vi "Calibration.vi"(7 "Show Front Panel":bool=TRUE, 8 "error in (no error)":errorcluster, 11 "file path (dialog if empty)":path=path "C:/work/Calibration.csv") -> (0 "error out":errorcluster, 3 "OutputData":string[][](array[string]))   [LabVIEW 2014]
uses:
  Type Definitions/HEWH Calibration.ctl
  Type Definitions/HEWH CalibrationTime.ctl
  Type Definitions/HEWH Calibration_SN.ctl
  Support VIs/CALIBRATION Equipment.vi
  <vilib>/Utility/file.llb/Write To Spreadsheet File (string).vi
panel:
  out "concatenated string":string
  out "snta":string[](array[string])
  in  "Tab Control":enum32{"Calibration Dates", "File Location"}(tab)
  in  "Equipment Description":T1
  in  "Manufacturer":T1
  in  "Model Number":T1
  in  "Calibration ID":T1
  in  "Complete":bool
  in  "Serial Number":T2
  in  "Last Calibrated":T3 {"Eq20" format="%<%x>T"; "Eq19" format="%<%x>T"; "Eq18" format="%<%x>T"; "Eq17" format="%<%x>T"; "Eq16" format="%<%x>T"; "Eq15" format="%<%x>T"; "Eq14" format="%<%x>T"; "Eq13" format="%<%x>T"; "Eq12" format="%<%x>T"; "Eq11" format="%<%x>T"; "Eq10" format="%<%x>T"; "Eq9" format="%<%x>T"; "Eq8" format="%<%x>T"; "Eq7" format="%<%x>T"; "Eq6" format="%<%x>T"; "Eq5" format="%<%x>T"; "Eq4" format="%<%x>T"; "Eq3" format="%<%x>T"; "Eq2" format="%<%x>T"; "Eq1" format="%<%x>T"}
  in  "Calibration Due":T3 {"Eq20" format="%<%x>T"; "Eq19" format="%<%x>T"; "Eq18" format="%<%x>T"; "Eq17" format="%<%x>T"; "Eq16" format="%<%x>T"; "Eq15" format="%<%x>T"; "Eq14" format="%<%x>T"; "Eq13" format="%<%x>T"; "Eq12" format="%<%x>T"; "Eq11" format="%<%x>T"; "Eq10" format="%<%x>T"; "Eq9" format="%<%x>T"; "Eq8" format="%<%x>T"; "Eq7" format="%<%x>T"; "Eq6" format="%<%x>T"; "Eq5" format="%<%x>T"; "Eq4" format="%<%x>T"; "Eq3" format="%<%x>T"; "Eq2" format="%<%x>T"; "Eq1" format="%<%x>T"}
  in  "Size":i32=20
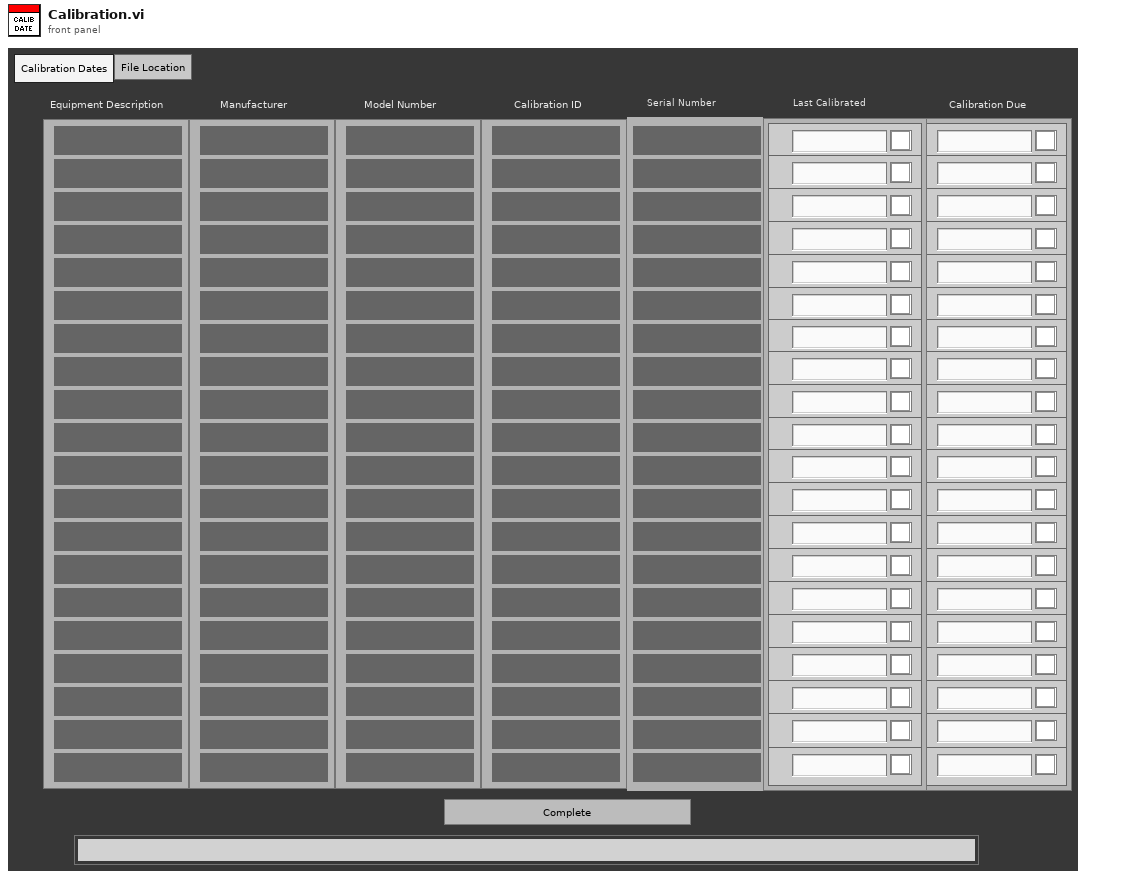
[diagram p1: front panel]
types:
  T1 = typedef "HEWH Calibration.ctl" = cluster{"Eq 1":string, "Eq 2":string, "Eq 3":string, "Eq 4":string, "Eq 5":string, "Eq 6":string, "Eq 7":string, "Eq 8":string, "Eq 9":string, "Eq 10":string, "Eq 11":string, "Eq 12":string, "Eq 13":string, "Eq 14":string, "Eq 15":string, "Eq 16":string, "Eq 17":string, "Eq 18":string, "Eq 19":string, "Eq 20":string}
  T2 = typedef "HEWH Calibration_SN.ctl" = cluster{"Eq 1":string, "Eq 2":string, "Eq 3":string, "Eq 4":string, "Eq 5":string, "Eq 6":string, "Eq 7":string, "Eq 8":string, "Eq 9":string, "Eq 10":string, "Eq 11":string, "Eq 12":string, "Eq 13":string, "Eq 14":string, "Eq 15":string, "Eq 16":string, "Eq 17":string, "Eq 18":string, "Eq 19":string, "Eq 20":string}
  T3 = typedef "HEWH CalibrationTime.ctl" = cluster{"Eq1":timestamp, "Eq2":timestamp, "Eq3":timestamp, "Eq4":timestamp, "Eq5":timestamp, "Eq6":timestamp, "Eq7":timestamp, "Eq8":timestamp, "Eq9":timestamp, "Eq10":timestamp, "Eq11":timestamp, "Eq12":timestamp, "Eq13":timestamp, "Eq14":timestamp, "Eq15":timestamp, "Eq16":timestamp, "Eq17":timestamp, "Eq18":timestamp, "Eq19":timestamp, "Eq20":timestamp}
  T4 = cluster{"Calibration Due":T3, "Last Calibrated":T3, "Serial Number":T2, "Calibration ID":T1, "Model Number":T1, "Manufacturer":T1, "Equipment Description":T1, i32}
  T5 = enum32{"invalid app kind", "Development System", "Run Time System", "Student Edition", "Embedded LabVIEW", "Evaluation", "Custom"}
  T6 = enum32{"Invalid", "Standard", "Closed", "Hidden", "Minimized", "Maximized"}
  T7 = cluster{"Core":cluster{"Current VI Reference":refnum<vi>, "Close Panel on Exit?":bool}, "Calibration Due":T3, "file path (dialog if empty)":path, "Serial Number":T2, "Calibration ID":T1, "Total Array":string[][], "Size":i32, "Last Calibrated":T3, "Model Number":T1, "Manufacturer":T1, "Equipment Description":T1}
  T8 = cluster{"Current VI Reference":refnum<vi>, "Close Panel on Exit?":bool}
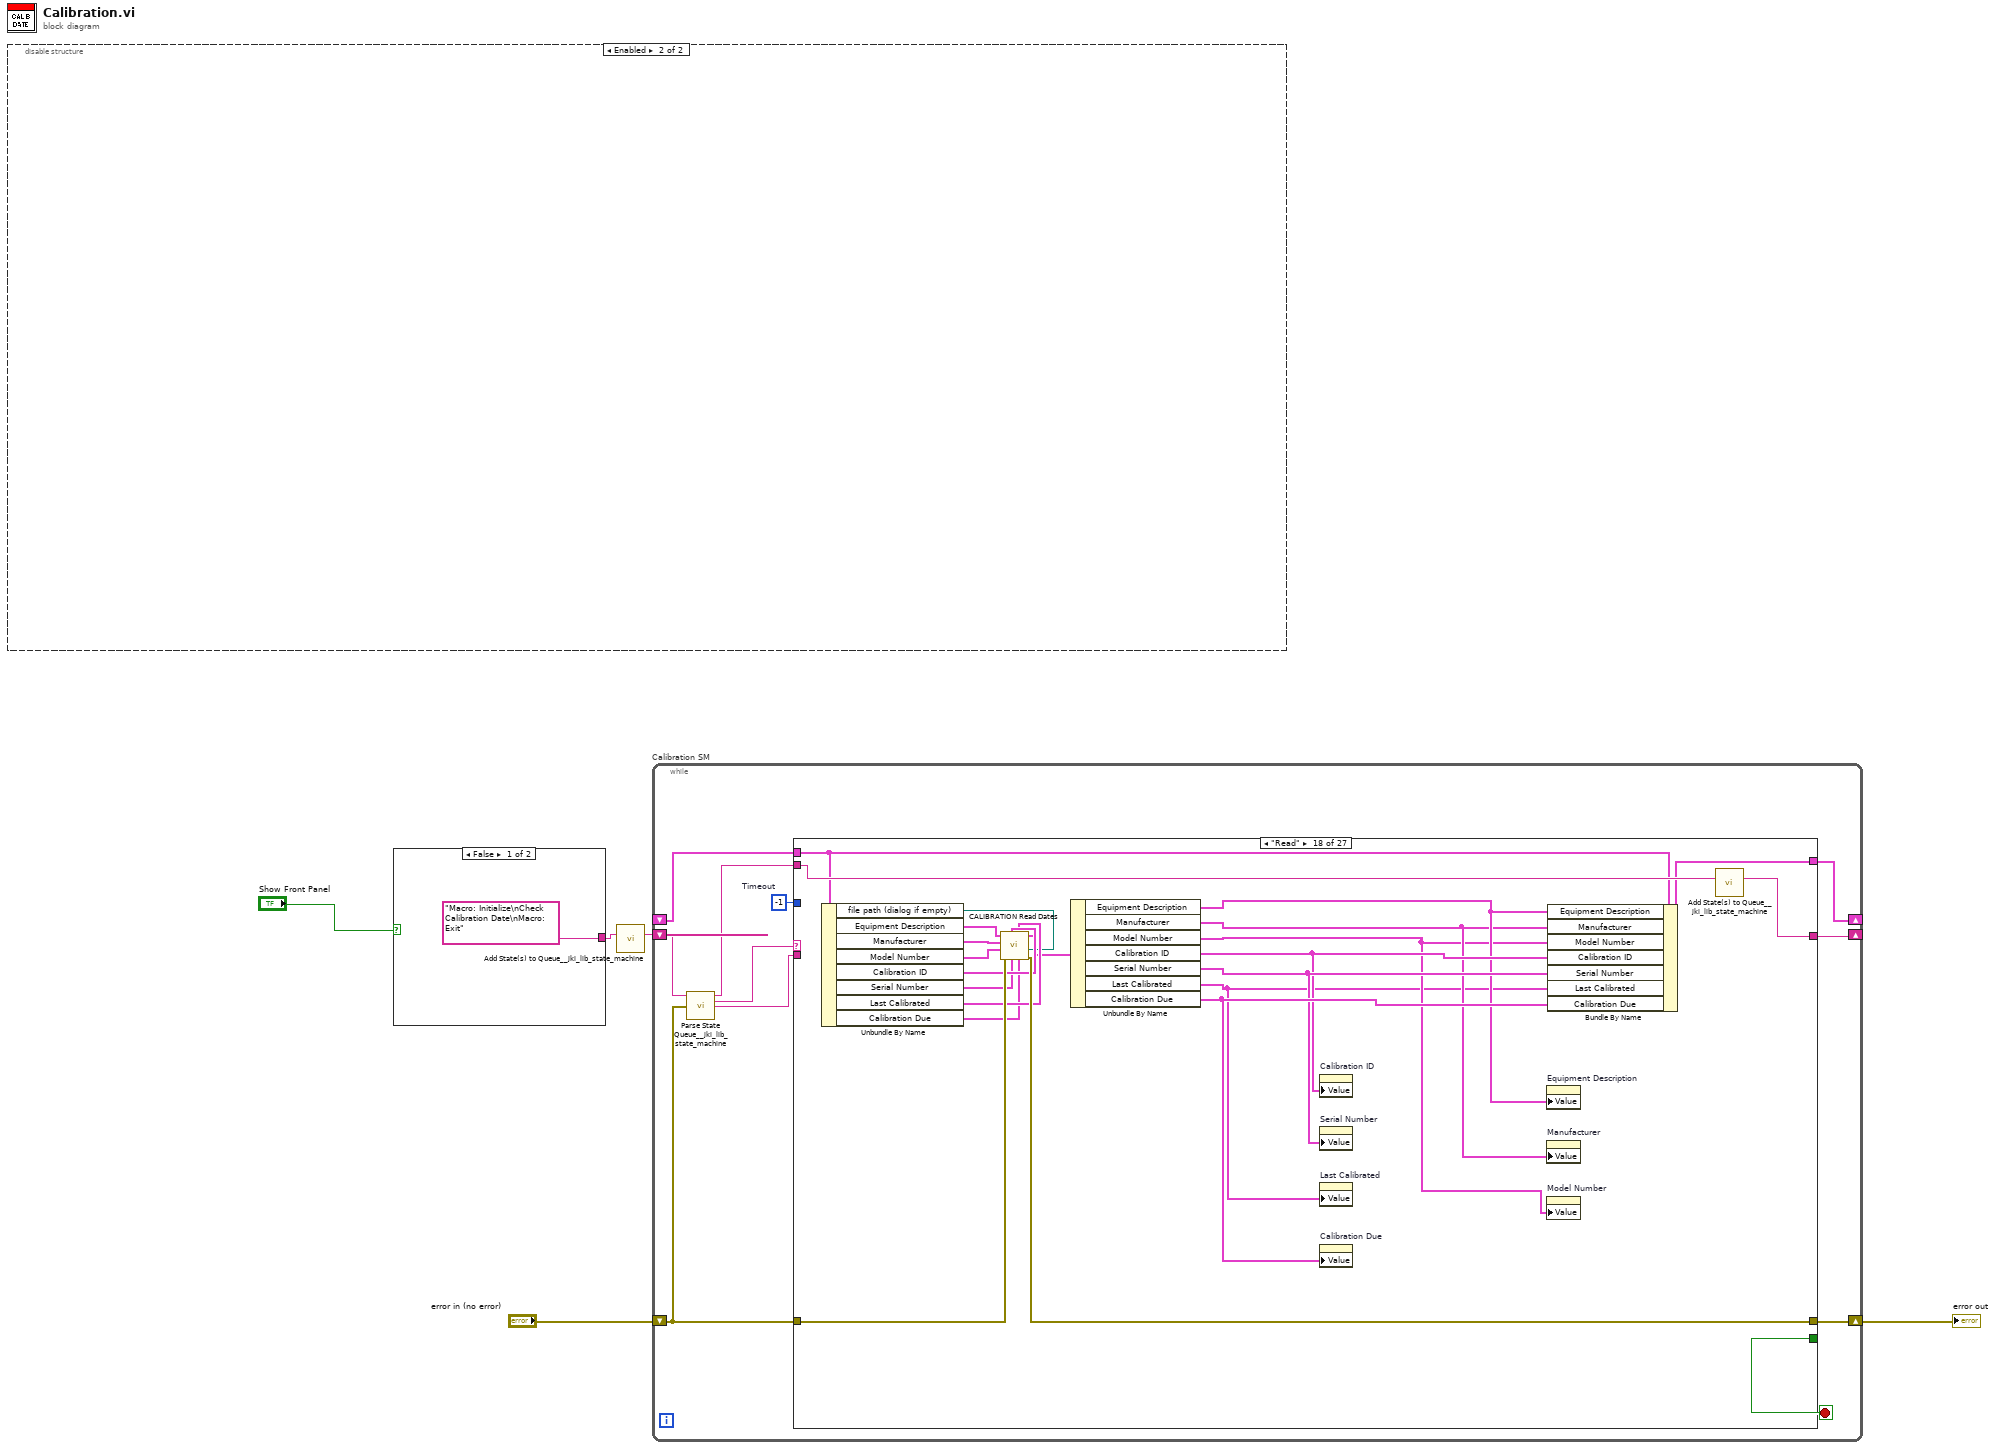
[diagram p0: block diagram]
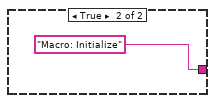
[diagram p2: hidden frame]
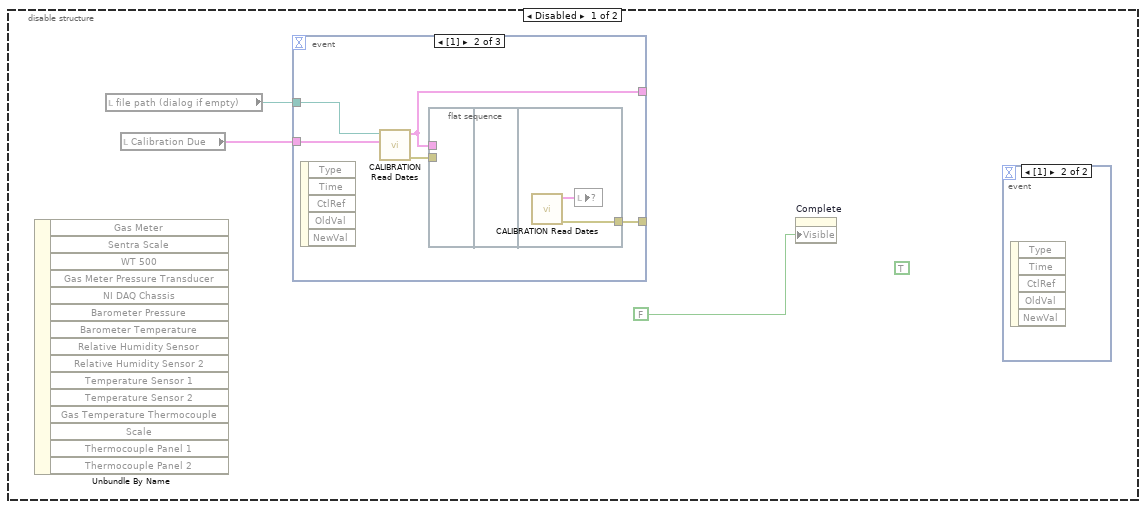
[diagram p3: hidden frame]
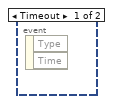
[diagram p4: hidden frame]
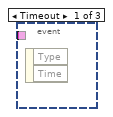
[diagram p5: hidden frame]
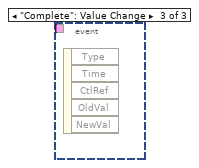
[diagram p6: hidden frame]
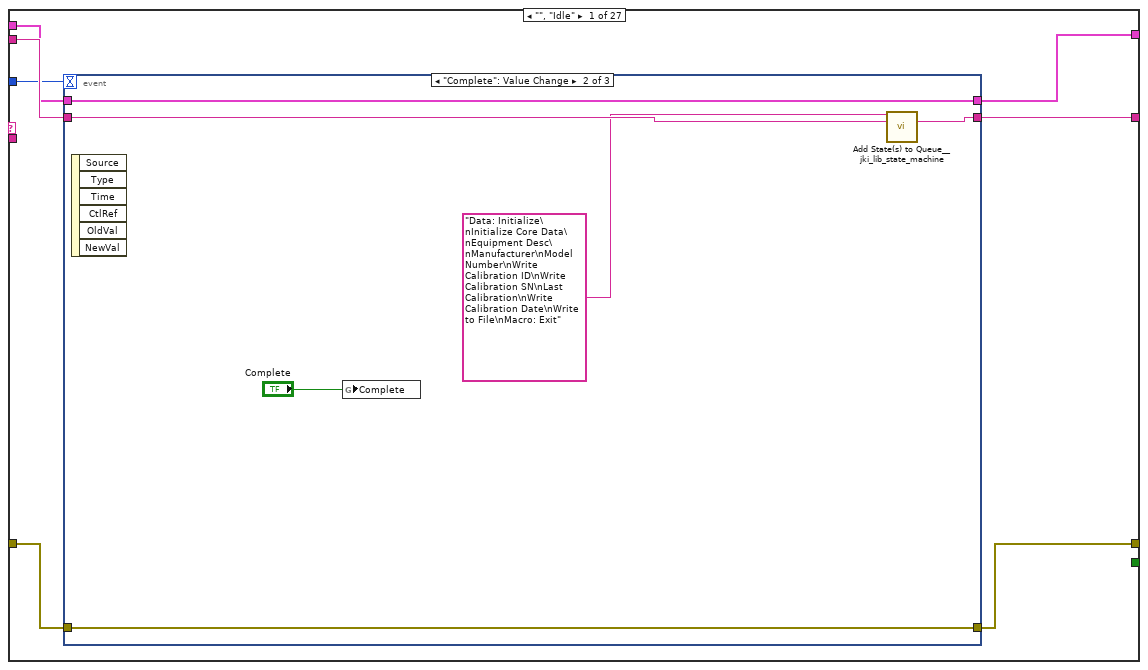
[diagram p7: hidden frame]
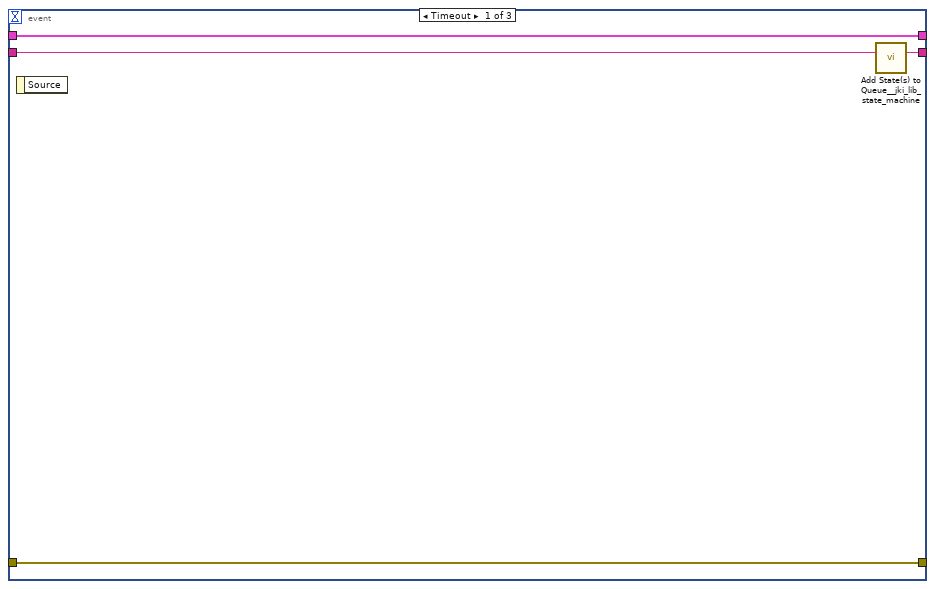
[diagram p8: hidden frame]
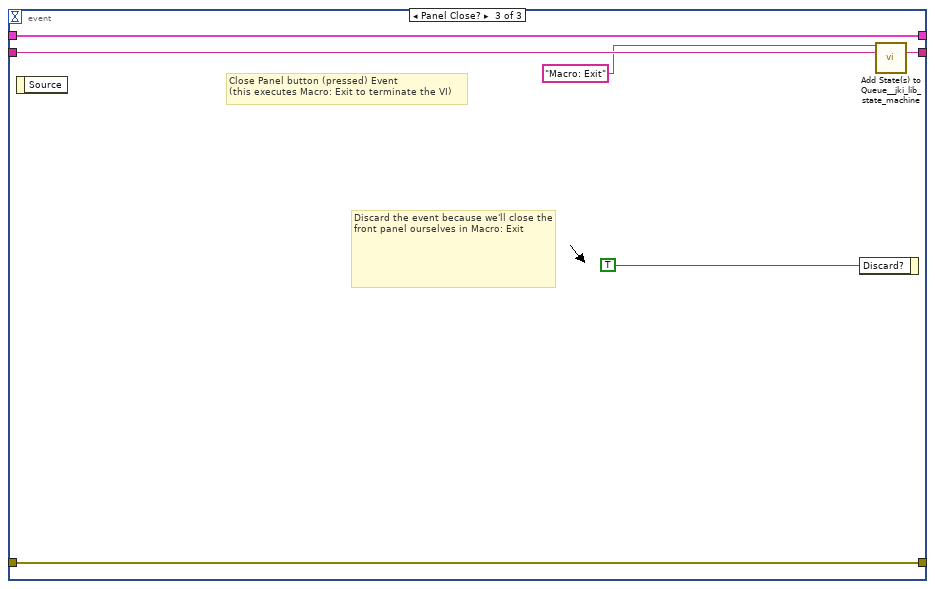
[diagram p9: hidden frame]
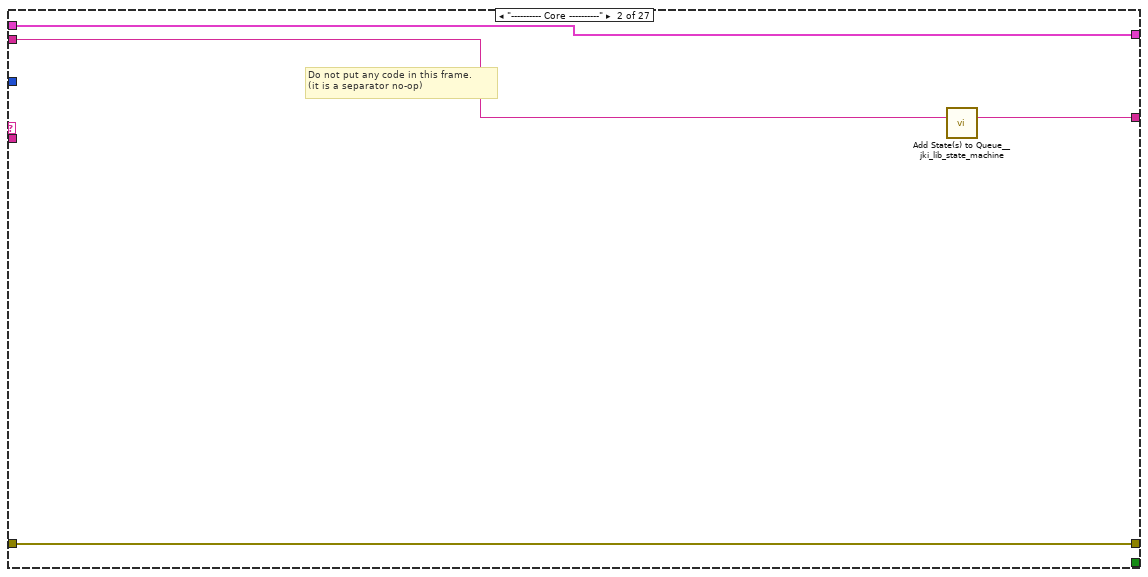
[diagram p10: hidden frame]
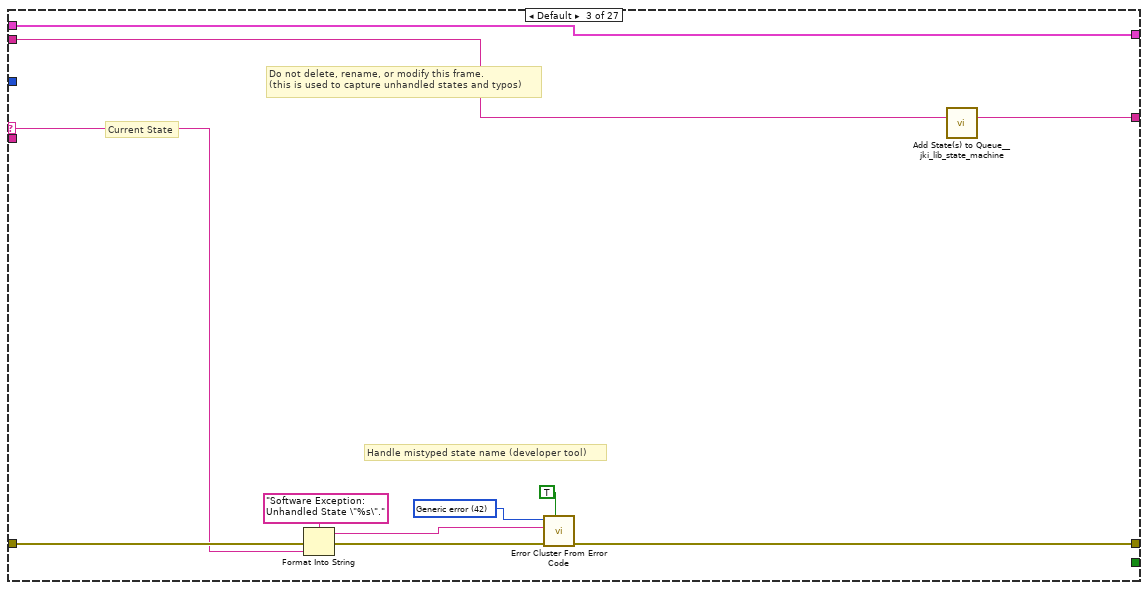
[diagram p11: hidden frame]
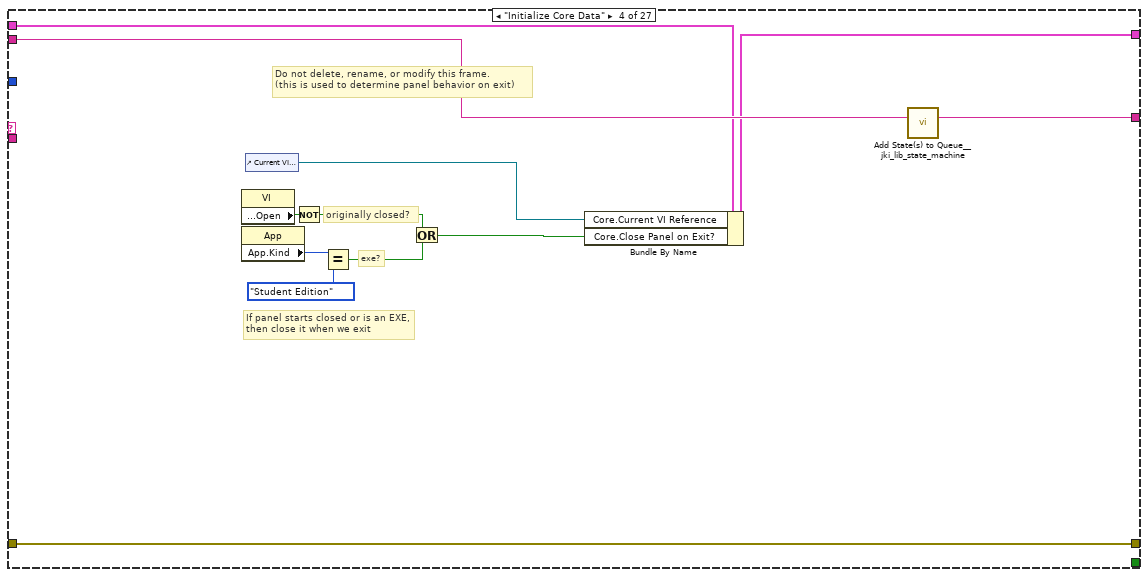
[diagram p12: hidden frame]
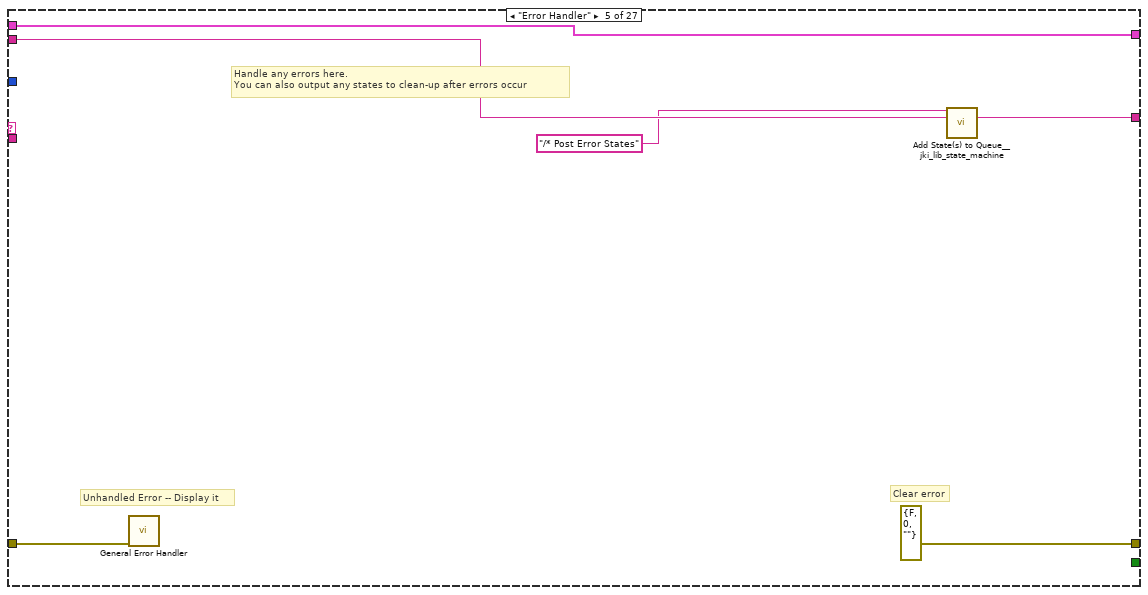
[diagram p13: hidden frame]
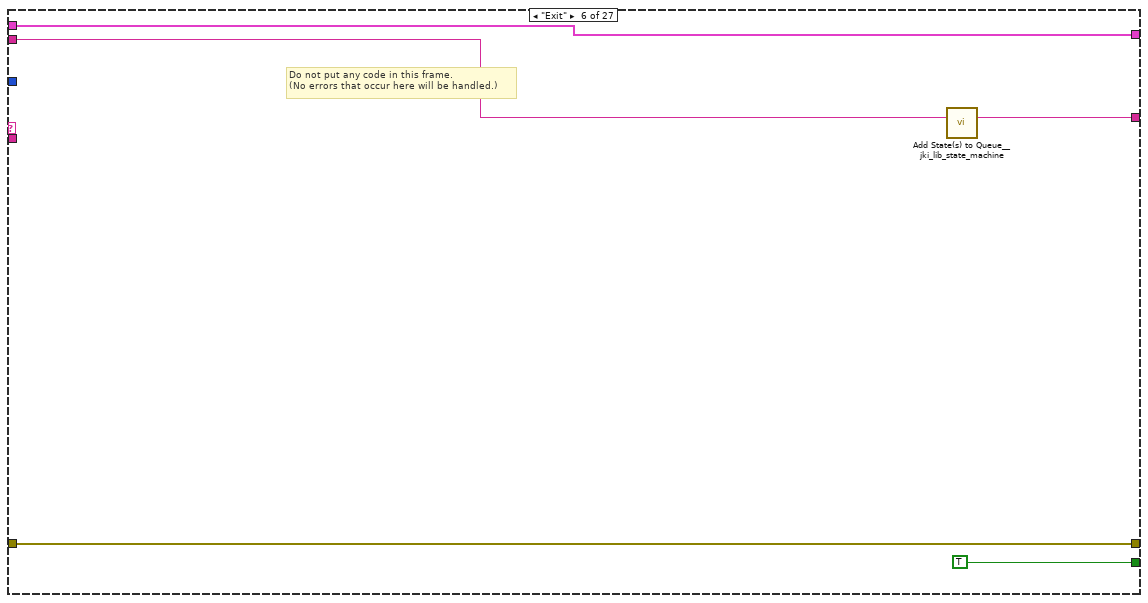
[diagram p14: hidden frame]
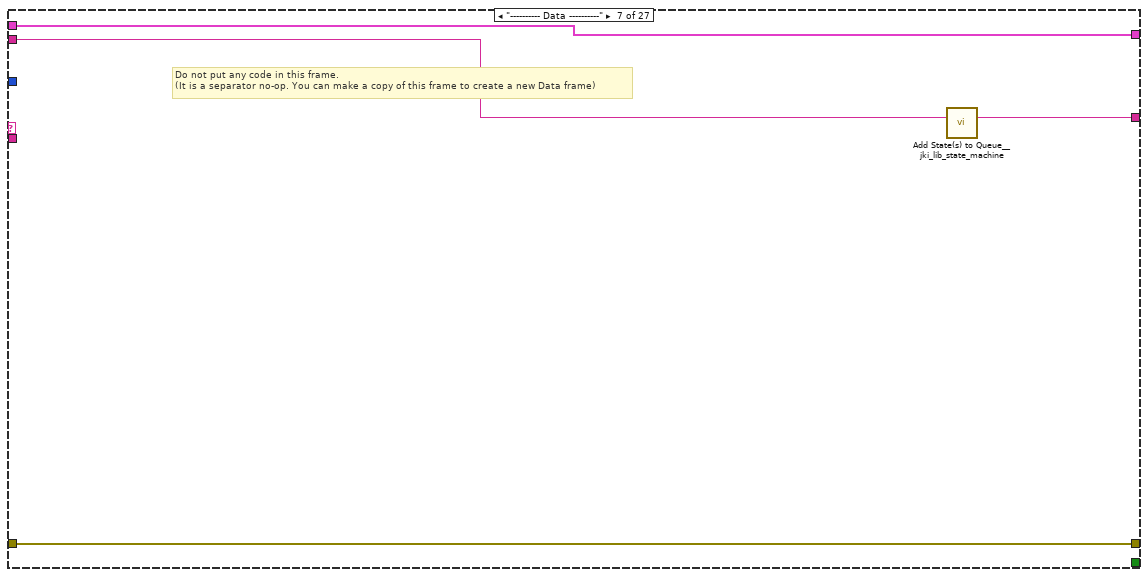
[diagram p15: hidden frame]
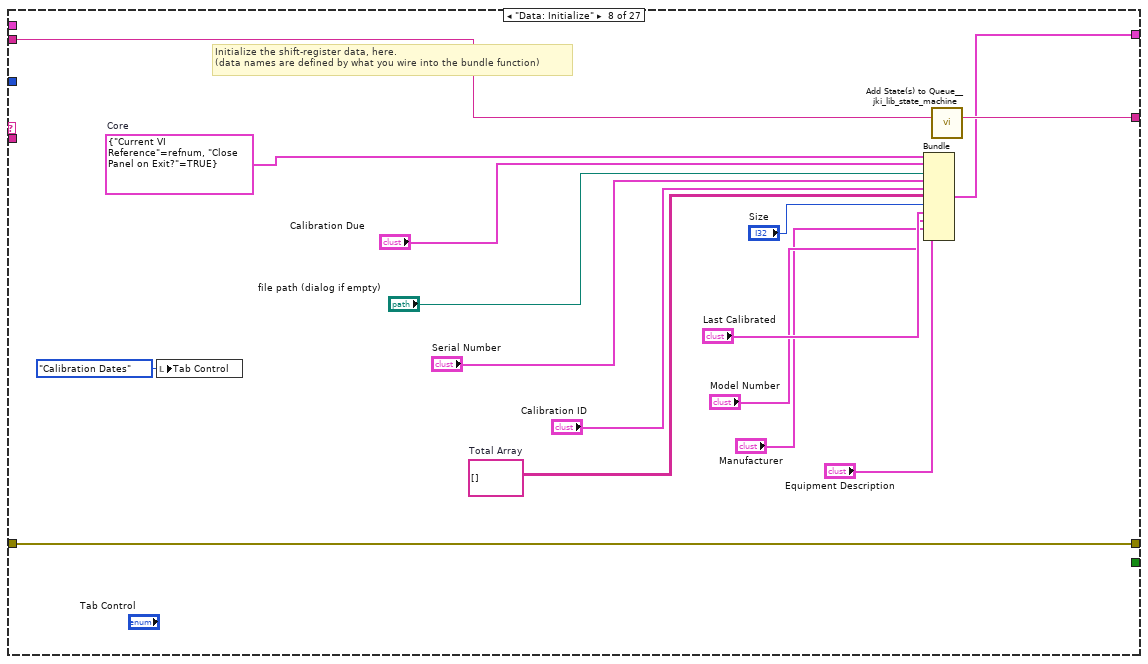
[diagram p16: hidden frame]
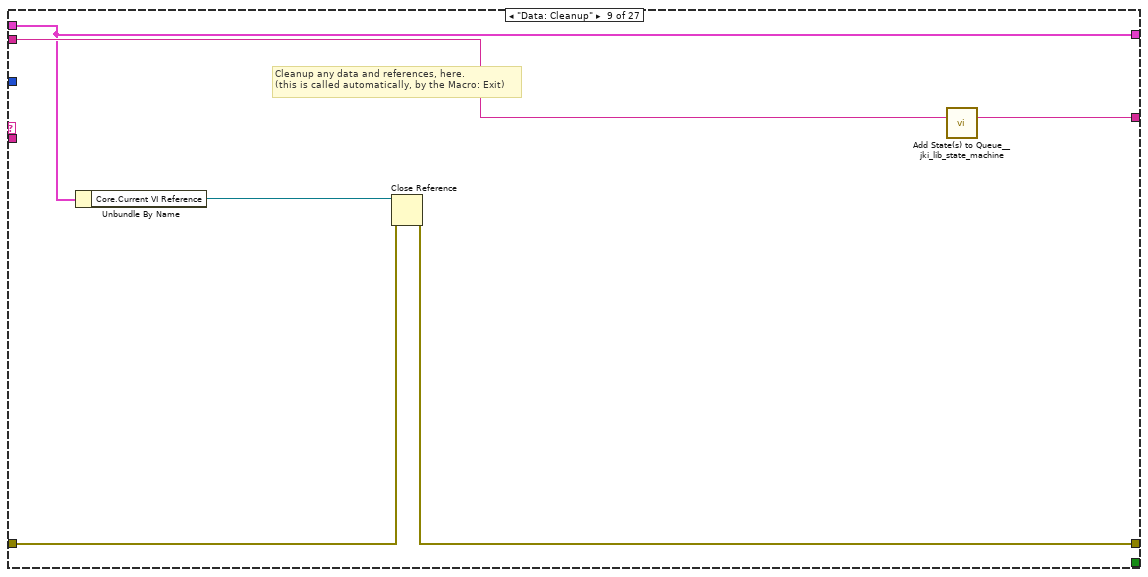
[diagram p17: hidden frame]
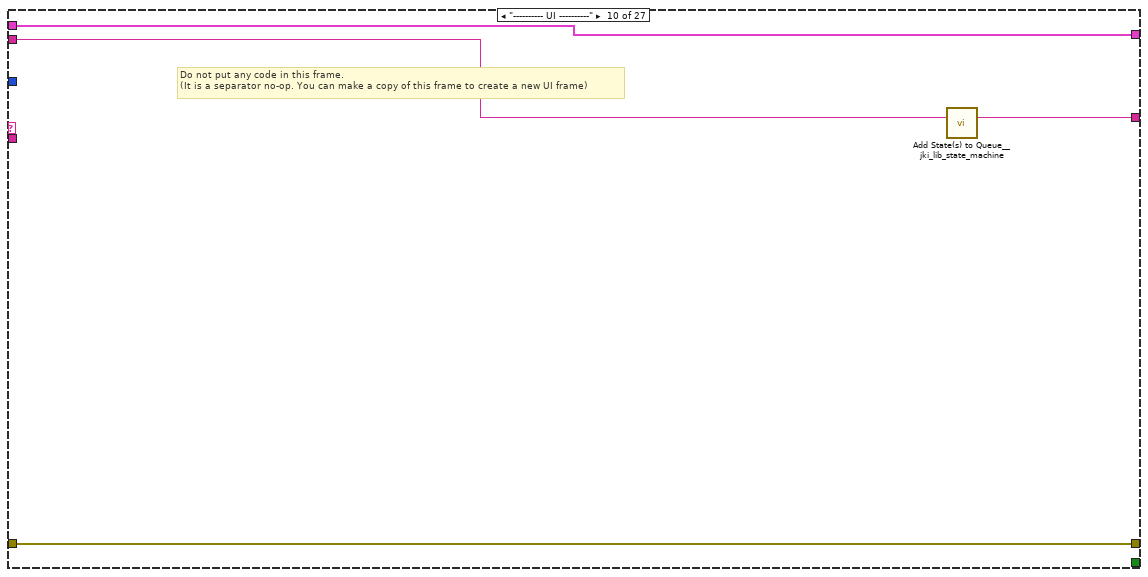
[diagram p18: hidden frame]
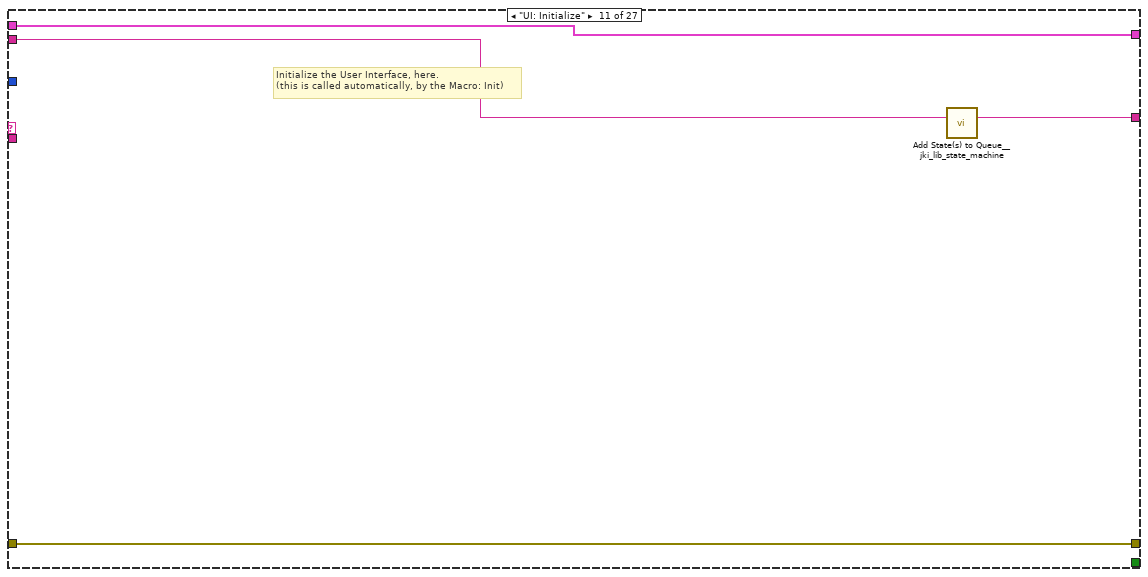
[diagram p19: hidden frame]
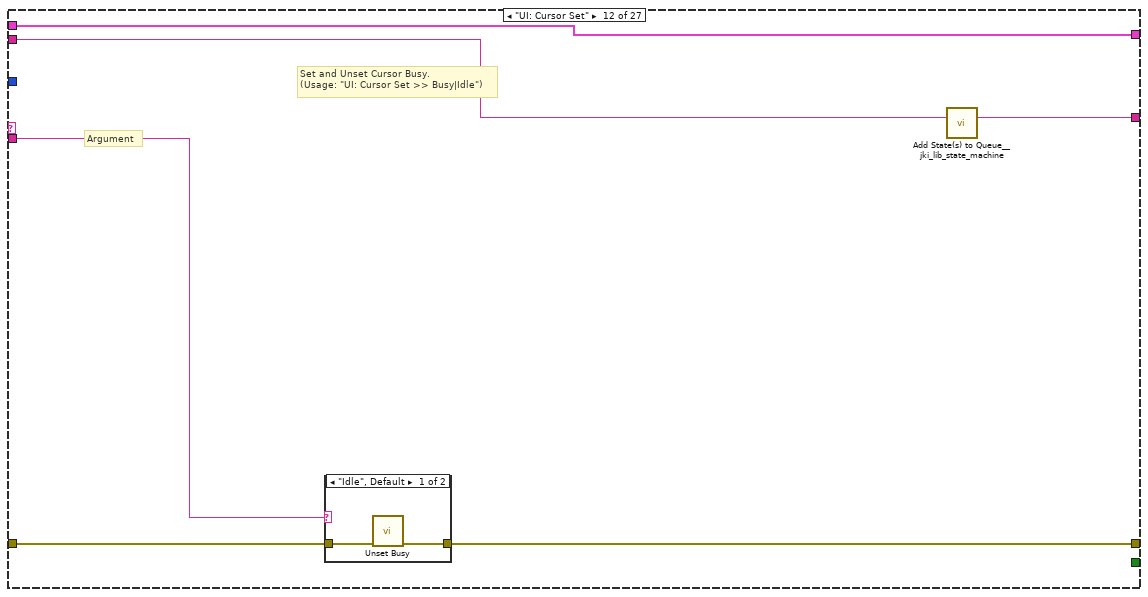
[diagram p20: hidden frame]
diagram:
  n1 = disable-structure shown="Enabled" {
    frame Disabled {
      w8 = TRUE ("Visible")
      n2 = Unbundle By Name() -> ()  [unwired: 1 in, 15 out]
      n3 = local read "file path (dialog if empty)"() -> (w6:path)
      n4 = local read "Calibration Due"() -> (w7:T3)
      n5 = event shown="[1]" {
        selector: _ -> [_ _ _]
        dyn-events: _ -> [_ _ _]
        timeout: _ -> [_ _ _]
        tunnel: [_ w12 _] -> _
        tunnel: [_ w15 _] -> _
        tunnel: w7 -> [_ w14 _]
        tunnel: w6 -> [_ w13 _]
        event Timeout {
          n6 = event-data() -> ()  [unwired: 1 in, 2 out]
        }
        event #1 (no event record) {
          n7 = event-data() -> ()  [unwired: 1 in, 5 out]
          n8 = call "CALIBRATION Read Dates.vi"("Manufacturer"=w14, "Equipment Description"=w13) -> ("error out"=w11:errorcluster, "output cluster"=w12:T4)  [unwired: 8 in]
          n9 = flat-sequence {
            tunnel: w11 -> [_]
            tunnel: w12 -> [_]
            tunnel: [w16] -> w15
            frame #0 {
            }
            frame #1 {
            }
            frame #2 {
              n10 = call "CALIBRATION Read Dates.vi"() -> ("error out"=w16:errorcluster, "output cluster"=w17:T4)  [unwired: 10 in]
              n11 = local write item#-1(w17) -> ()
            }
          }
        }
        event "Complete": Value Change {
          n12 = event-data() -> ()  [unwired: 1 in, 5 out]
        }
      }
      n13 = property on="Complete" class="Bool"("Visible"=FALSE) -> (error out=w9:errorcluster)  [unwired: 2 in, 1 out]
      n14 = event shown="[1]" {
        selector: _ -> [_ _]
        dyn-events: _ -> [_ _]
        timeout: _ -> [_ _]
        event Timeout {
          n15 = event-data() -> ()  [unwired: 1 in, 2 out]
        }
        event #1 (no event record) {
          n16 = event-data() -> ()  [unwired: 1 in, 5 out]
        }
      }
    }
    frame Enabled {
    }
  }
  n17 = case shown="False" "Show Front Panel" {
    tunnel: ["Macro: Initialize\nCheck Calibration Date\nMacro: Exit" "Macro: Initialize"] -> w4
    frame False {
    }
    frame True {
    }
  }
  n18 = call <vilib>:"Add State(s) to Queue__jki_lib_state_machine.vi"("State(s) in (\"\")"=w4) -> ("States Out"=w5:string)  [unwired: 14 in]
  n19 = while "Calibration SM" {
    shift-right: [w23] -> _
    shift-left: _ -> [w22]
    shift-right: [w26] -> w2
    shift-left: "error in (no error)" -> [w20]
    shift-right: [w25] -> _
    shift-left: w5 -> [w27]
    stop <- w24 stop-if-true
    w21 = -1  # Timeout
    n20 = call <vilib>:"Parse State Queue__jki_lib_state_machine.vi"("State Queue"=w27, "Error In (no error)"=w20) -> ("Remaining States"=w29:string, "Current State"=w30:string, "Arguments"=w28:string)  [unwired: 11 in]
    n21 = case shown="\"Read\"" w30 {
      selector: w30 -> [_ _ w58 _ _ _ _ _ _ _ _ _ _ _ _ _ _ _ _ _ _ _ _ _ _ _ _]
      tunnel: w29 -> [w37 w57 w62 w80 w86 w91 w95 w111 w117 w121 w125 w131 w142 w168 w173 w183 w187 w209 w220 w381 w441 w501 w561 w621 w681 w763 w841]
      tunnel: w28 -> [_ _ _ _ _ _ _ _ _ _ _ w126 w136 _ _ _ _ _ _ _ _ _ _ _ _ _ _]
      tunnel: w22 -> [w35 w54 w60 w71 w83 w89 w92 _ w112 w118 w123 w129 w138 w165 w170 w180 w184 w207 w218 w375 w435 w495 w555 w615 w674 w756 w839]
      tunnel: [w34 w55 w64 w77 errorcluster {"status"=FALSE, "code"=0, "source"=""} ("error out") w88 w93 w108 w113 w119 w122 w127 w139 w166 w171 w181 w185 w204 w217 w376 w436 w496 w556 w616 w676 w758 w836] -> w26
      tunnel: w20 -> [w33 w55 w63 w77 w82 w88 w93 w108 w114 w119 w122 w128 w140 w166 w171 w181 w185 w205 w217 w377 w437 w497 w557 w617 w677 w759 w836]
      tunnel: [w36 w56 w61 w79 w85 w90 w94 w110 w116 w120 w124 w130 w141 w167 w172 w182 w186 w208 w219 w380 w440 w500 w560 w620 w680 w762 w840] -> w25
      tunnel: [_ _ _ _ _ TRUE _ _ _ _ _ _ _ _ _ _ _ _ _ _ _ _ _ _ _ _ _] -> w24
      tunnel: [w32 w54 w60 w78 w83 w89 w92 w109 w112 w118 w123 w129 w138 w165 w170 w180 w184 w206 w218 w374 w434 w494 w554 w614 w673 w755 w839] -> w23
      tunnel: w21 -> [w31 _ _ _ _ _ _ _ _ _ _ _ _ _ _ _ _ _ _ _ _ _ _ _ _ _ _]
      frame "", "Idle" {
        n22 = event shown="[1] \"Complete\": Value Change" {
          selector: _ -> [_ _ _]
          dyn-events: _ -> [_ _ _]
          timeout: w31 -> [_ _ _]
          tunnel: w37 -> [w41 w46 w53]
          tunnel: [w40 w47 w52] -> w36
          tunnel: w35 -> [w38 w43 w50]
          tunnel: [w39 w45 w51] -> w34
          tunnel: w33 -> [w39 w45 w51]
          tunnel: [w38 w43 w50] -> w32
          event Timeout {
            n23 = event-data() -> ()  [unwired: 1 in, 1 out]
            n24 = call <vilib>:"Add State(s) to Queue__jki_lib_state_machine.vi"("State(s) in (\"\")"=w41) -> ("States Out"=w40:string)  [unwired: 14 in]
          }
          event "Complete": Value Change {
            n25 = event-data() -> ()  [unwired: 1 in, 6 out]
            n26 = global write "CALIBRATION Equipment.vi" "Complete"("Complete") -> ()
            n27 = call <vilib>:"Add State(s) to Queue__jki_lib_state_machine.vi"("State(s) in Front (\"\")"="Data: Initialize\nInitialize Core Data\nEquipment Desc\nManufacturer\nModel Number\nWrite Calibration ID\nWrite Calibration SN\nLast Calibration\nWrite Calibration Date\nWrite to File\nMacro: Exit", "State(s) in (\"\")"=w46) -> ("States Out"=w47:string)  [unwired: 13 in]
          }
          event Panel Close? {
            # "Discard the event because we'll close the front panel ourselves in Macro: Exit"
            # "Close Panel button (pressed) Event\n(this executes Macro: Exit to terminate the VI)"
            n28 = event-data() -> ()  [unwired: 1 in, 1 out]
            n29 = event-data("Discard?"=TRUE) -> ()  [unwired: 1 in, 1 out]
            n30 = call <vilib>:"Add State(s) to Queue__jki_lib_state_machine.vi"("State(s) in Front (\"\")"="Macro: Exit", "State(s) in (\"\")"=w53) -> ("States Out"=w52:string)  [unwired: 13 in]
          }
        }
      }
      frame "---------- Core ----------" {
        # "Do not put any code in this frame.\n(it is a separator no-op)"
        n31 = call <vilib>:"Add State(s) to Queue__jki_lib_state_machine.vi"("State(s) in (\"\")"=w57) -> ("States Out"=w56:string)  [unwired: 14 in]
      }
      frame Default {
        w67 = 42 items=["No error", "Argument error", "Memory is full", "Out of zone", "End of file", "File already open", "Generic file I/O error", "File not found", "File permission error", "Disk is full", "Duplicate path", "Too many files open", "System feature not enabled", "Resource file not found", "Cannot add resource", "Resource not found", "Image not found", "Image memory error", "Pen does not exist", "Config type invalid", "Config token not found", "Config parse error", "Config memory error", "Bad external code format", "Bad external code offset", "External code not present", "Null window", "Destroy window error", "Null menu", "Print aborted", "Bad print record", "Print driver error", "Windows error during printing", "Memory error during printing", "Print dialog error", "Generic print error", "Invalid device refnum", "Device not found", "Device parameter error", "Device unit error", "Cannot open device", "Device call aborted", "Generic error", "Cancelled by user", "Object ID too low", "Object ID too high", "Object not in heap", "Unknown heap", "Unknown object (invalid DefProc)", "Unknown object (DefProc not in table)", "Message out of range", "Invalid (null) method", "Unknown message", "Manager call not supported", "Bad address", "Network operation in progress", "Network operation timed out", "Connection is busy", "Network attribute not supported", "Network error", "Address in use", "System out of memory", "Connection aborted", "Connection refused", "Not connected", "Already connected", "Connection closed", "Initialization error (interapplication manager)", "Bad occurrence", "Wait on unbound occurrence handler", "Occurrence queue overflow", "Datalog type conflict", "Unused", "Unrecognized type (interapplication manager)", "Memory corrupt", "Failed to make temporary DLL", "Old CIN version", "Drag socket not found", "Failed to load drop-object", "Failed to register OLE object", "Failed to release OLE object", "Format specifier type mismatch", "Unknown format specifier", "Too few format specifiers", "Too many format specifiers", "Scan failed", "Newer CIN version", "Error converting to variant", "Runtime menu error", "Password tampered", "Variant attribute not found", "Incompatible variant data type", "Event data is not available", "Event Store is not present", "Occurrence is not found", "Event Queue is not created", "Event info is not available", "Refnum passed is NULL", "Error retrieving Class GUID", "Error retrieving CoClass GUID", "Error retrieving TypeLib GUID.", "Bad built application magic bytes.", "Specific driver is different from the specific driver associated with the Logical Name.", "There is no session opened to the class driver.", "Max Error", "MAX - Error with config objects", "MAX - Error loading configuration", "MAX - Group not supported"]
        # "Current State"
        # "Do not delete, rename, or modify this frame.\n(this is used to capture unhandled states and typos)"
        # "Handle mistyped state name (developer tool)"
        n32 = Format Into String(format string="Software Exception: Unhandled State \"%s\"." ("message"), error in=w63, w58) -> (resulting string=w66:string, error out=w65:errorcluster)  [unwired: 1 in]
        n33 = call <vilib>:"Error Cluster From Error Code.vi"("show call chain? (False)"=TRUE, "error in (no error)"=w65, "error message (\"\")"=w66, "error code (0)"=w67) -> ("error out"=w64:errorcluster)  [unwired: 5 in]
        n34 = call <vilib>:"Add State(s) to Queue__jki_lib_state_machine.vi"("State(s) in (\"\")"=w62) -> ("States Out"=w61:string)  [unwired: 14 in]
      }
      frame "Initialize Core Data" {
        # "Do not delete, rename, or modify this frame.\n(this is used to determine panel behavior on exit)"
        # "originally closed?"
        # "exe?"
        # "If panel starts closed or is an EXE, then close it when we exit"
        n35 = property class="VI"() -> ("Front Panel.Open"=w76:bool)  [unwired: 2 in, 2 out]
        n36 = property class="App"() -> ("App.Kind"=w75:T5)  [unwired: 2 in, 2 out]
        n37 = control-ref of="Current VI Reference"() -> (w69:refnum<vi>)
        n38 = Not(x=w76) -> (.not. x?=w73:bool)
        n39 = Equal?(x=w75, y=T5."Student Edition" ("Application:Kind")) -> (x = y?=w72:bool)
        n40 = Or(x=w73, y=w72) -> (x .or. y?=w70:bool)
        n41 = Bundle By Name(cluster=w71, "Core.Current VI Reference"=w69, "Core.Close Panel on Exit?"=w70) -> (w78:T7)
        n42 = call <vilib>:"Add State(s) to Queue__jki_lib_state_machine.vi"("State(s) in (\"\")"=w80) -> ("States Out"=w79:string)  [unwired: 14 in]
      }
      frame "Error Handler" {
        # "Unhandled Error -- Display it"
        # "Handle any errors here.\nYou can also output any states to clean-up after errors occur"
        # "Clear error"
        n43 = call <vilib>:"General Error Handler.vi"("error in (no error)"=w82) -> ()  [unwired: 10 in, 5 out]
        n44 = call <vilib>:"Add State(s) to Queue__jki_lib_state_machine.vi"("State(s) in Front (\"\")"="/* Post Error States", "State(s) in (\"\")"=w86) -> ("States Out"=w85:string)  [unwired: 13 in]
      }
      frame "Exit" {
        # "Do not put any code in this frame.\n(No errors that occur here will be handled.)"
        n45 = call <vilib>:"Add State(s) to Queue__jki_lib_state_machine.vi"("State(s) in (\"\")"=w91) -> ("States Out"=w90:string)  [unwired: 14 in]
      }
      frame "---------- Data ----------" {
        # "Do not put any code in this frame.\n(It is a separator no-op. You can make a copy of this frame to create a new Data frame)"
        n46 = call <vilib>:"Add State(s) to Queue__jki_lib_state_machine.vi"("State(s) in (\"\")"=w95) -> ("States Out"=w94:string)  [unwired: 14 in]
      }
      frame "Data: Initialize" {
        w105 = string[][] []  # Total Array
        w107 = T8 {"Current VI Reference"=refnum, "Close Panel on Exit?"=TRUE}  # Core
        # "Initialize the shift-register data, here.\n(data names are defined by what you wire into the bundle function)"
        n47 = local write "Tab Control"(enum32{"Calibration Dates", "File Location"}."Calibration Dates" ("Tab Control")) -> ()
        n48 = Bundle("Core"=w107, "Calibration Due"="Calibration Due", "file path (dialog if empty)"="file path (dialog if empty)", "Serial Number"="Serial Number", "Calibration ID"="Calibration ID", "Total Array"=w105, "Size"="Size", "Last Calibrated"="Last Calibrated", "Model Number"="Model Number", "Manufacturer"="Manufacturer", "Equipment Description"="Equipment Description") -> (w109:T7)  [unwired: 1 in]
        n49 = call <vilib>:"Add State(s) to Queue__jki_lib_state_machine.vi"("State(s) in (\"\")"=w111) -> ("States Out"=w110:string)  [unwired: 14 in]
      }
      frame "Data: Cleanup" {
        # "Cleanup any data and references, here.\n(this is called automatically, by the Macro: Exit)"
        n50 = Unbundle By Name(w112) -> ("Core.Current VI Reference"=w115:refnum<vi>)
        n51 = Close Reference(reference=w115, error in (no error)=w114) -> (error out=w113:errorcluster)
        n52 = call <vilib>:"Add State(s) to Queue__jki_lib_state_machine.vi"("State(s) in (\"\")"=w117) -> ("States Out"=w116:string)  [unwired: 14 in]
      }
      frame "---------- UI ----------" {
        # "Do not put any code in this frame.\n(It is a separator no-op. You can make a copy of this frame to create a new UI frame)"
        n53 = call <vilib>:"Add State(s) to Queue__jki_lib_state_machine.vi"("State(s) in (\"\")"=w121) -> ("States Out"=w120:string)  [unwired: 14 in]
      }
      frame "UI: Initialize" {
        # "Initialize the User Interface, here.\n(this is called automatically, by the Macro: Init)"
        n54 = call <vilib>:"Add State(s) to Queue__jki_lib_state_machine.vi"("State(s) in (\"\")"=w125) -> ("States Out"=w124:string)  [unwired: 14 in]
      }
      frame "UI: Cursor Set" {
        # "Argument"
        # "Set and Unset Cursor Busy.\n(Usage: \"UI: Cursor Set >> Busy|Idle\")"
        n55 = case shown="\"Idle\", Default" w126 {
          tunnel: w128 -> [w133 w135]
          tunnel: [w132 w134] -> w127
          frame "Idle", Default {
            n56 = call <vilib>:"Unset Busy.vi"("error in (no error)"=w133) -> ("error out"=w132:errorcluster)  [unwired: 10 in]
          }
          frame "Busy" {
            n57 = call <vilib>:"Set Busy.vi"("error in (no error)"=w135) -> ("error out"=w134:errorcluster)  [unwired: 9 in, 1 out]
          }
        }
        n58 = call <vilib>:"Add State(s) to Queue__jki_lib_state_machine.vi"("State(s) in (\"\")"=w131) -> ("States Out"=w130:string)  [unwired: 14 in]
      }
      frame "UI: Front Panel State" {
        # "Argument"
        # "Set Front Panel Open or Closed\n(Usage: \"UI: Front Panel State >> Open|Close\")"
        n59 = Unbundle By Name(w138) -> ("Core.Current VI Reference"=w137:refnum<vi>)
        n60 = case shown="\"Open\", Default" w136 {
          tunnel: w140 -> [w146 w159]
          tunnel: [w148 w160] -> w139
          tunnel: w137 -> [w147 w157]
          frame "Open", Default {
            n61 = property class="VI"(reference=w147, error in=w146) -> (reference out=w144:refnum<vi>, error out=w145:errorcluster, "Front Panel.Open"=w143:bool)
            n62 = case shown="True" w143 {
              tunnel: [w151 w154] -> w148
              tunnel: w145 -> [w150 w154]
              tunnel: w144 -> [w149 _]
              frame False {
                n63 = invoke class="VI" method="FP.Open"(reference=w149, error in=w150, "Activate"=TRUE, "State"=T6."Standard") -> (error out=w151:errorcluster)  [unwired: 1 in, 4 out]
              }
              frame True {
              }
            }
          }
          frame "Close" {
            n64 = property class="VI"(reference=w157, error in=w159) -> (reference out=w156:refnum<vi>, error out=w158:errorcluster, "Front Panel.Open"=w155:bool)
            n65 = case shown="True" w155 {
              tunnel: [w161 w164] -> w160
              tunnel: w158 -> [w161 w163]
              tunnel: w156 -> [_ w162]
              frame False {
              }
              frame True {
                n66 = invoke class="VI" method="FP.Close"(reference=w162, error in=w163) -> (error out=w164:errorcluster)  [unwired: 1 in, 2 out]
              }
            }
          }
        }
        n67 = call <vilib>:"Add State(s) to Queue__jki_lib_state_machine.vi"("State(s) in (\"\")"=w142) -> ("States Out"=w141:string)  [unwired: 14 in]
      }
      frame "---------- Macro ----------" {
        # "Do not put any code in this frame.\n(It is a separator no-op. You can make a copy of this frame to create a new Macro frame)"
        n68 = call <vilib>:"Add State(s) to Queue__jki_lib_state_machine.vi"("State(s) in (\"\")"=w168) -> ("States Out"=w167:string)  [unwired: 14 in]
      }
      frame "Macro: Initialize" {
        w169 = "Data: Initialize\nInitialize Core Data\nUI: Initialize\nUI: Front Panel State >> Open\nRead\nCheck Calibration Date"  # Data: Initialize Initialize Core Data UI: Initialize UI: Front Panel State >> Open Read Check Calibration Date
        # "Initialization Macro\n(This is called once, when the VI starts)"
        n69 = call <vilib>:"Add State(s) to Queue__jki_lib_state_machine.vi"("State(s) in Front (\"\")"=w169, "State(s) in (\"\")"=w173) -> ("States Out"=w172:string)  [unwired: 13 in]
      }
      frame "Macro: Exit" {
        # "Exit Macro\n(This is called once, when the VI exits)"
        n70 = Unbundle By Name(w180) -> ("Core.Close Panel on Exit?"=w179:bool)
        n71 = Select(t="UI: Front Panel State >> Close", s=w179, f="") -> (s? t:f=w176:string)
        n72 = call <vilib>:"Add State(s) to Queue__jki_lib_state_machine.vi"("State(s) in (\"\")"=w176, "State(s) at Back (\"\")"="Data: Cleanup\nExit") -> ("States Out"=w174:string)  [unwired: 13 in]
        n73 = call <vilib>:"Add State(s) to Queue__jki_lib_state_machine.vi"("State(s) in Front (\"\")"=w174, "State(s) in (\"\")"=w183) -> ("States Out"=w182:string)  [unwired: 13 in]
      }
      frame "---------- New Category ----------" {
        # "Template Separator\n(You can make a copy of, or modify, this frame)"
        n74 = call <vilib>:"Add State(s) to Queue__jki_lib_state_machine.vi"("State(s) in (\"\")"=w187) -> ("States Out"=w186:string)  [unwired: 14 in]
      }
      frame "Read" {
        n75 = Unbundle By Name(w207) -> ("file path (dialog if empty)"=w196:path, "Equipment Description"=w203:T1, "Manufacturer"=w202:T1, "Model Number"=w201:T1, "Calibration ID"=w200:T1, "Serial Number"=w199:T2, "Last Calibrated"=w198:T3, "Calibration Due"=w197:T3)
        n76 = call "CALIBRATION Read Dates.vi"("File Path"=w196, "Calibration Due"=w197, "Last Calibrated"=w198, "Serial Number"=w199, "Calibration ID"=w200, "error in (no error)"=w205, "Model Number"=w201, "Manufacturer"=w202, "Equipment Description"=w203) -> ("error out"=w204:errorcluster, "output cluster"=w195:T4)  [unwired: 1 in]
        n77 = Unbundle By Name(w195) -> ("Equipment Description"=w191:T1, "Manufacturer"=w190:T1, "Model Number"=w189:T1, "Calibration ID"=w192:T1, "Serial Number"=w193:T2, "Last Calibrated"=w188:T3, "Calibration Due"=w194:T3)
        n78 = property on="Calibration ID" class="Clust (strict)"("Value"=w192) -> ()  [unwired: 2 in, 2 out]
        n79 = property on="Serial Number" class="Clust (strict)"("Value"=w193) -> ()  [unwired: 2 in, 2 out]
        n80 = property on="Last Calibrated" class="Clust (strict)"("Value"=w188) -> ()  [unwired: 2 in, 2 out]
        n81 = property on="Calibration Due" class="Clust (strict)"("Value"=w194) -> ()  [unwired: 2 in, 2 out]
        n82 = property on="Equipment Description" class="Clust (strict)"("Value"=w191) -> ()  [unwired: 2 in, 2 out]
        n83 = property on="Manufacturer" class="Clust (strict)"("Value"=w190) -> ()  [unwired: 2 in, 2 out]
        n84 = property on="Model Number" class="Clust (strict)"("Value"=w189) -> ()  [unwired: 2 in, 2 out]
        n85 = Bundle By Name(cluster=w207, "Equipment Description"=w191, "Manufacturer"=w190, "Model Number"=w189, "Calibration ID"=w192, "Serial Number"=w193, "Last Calibrated"=w188, "Calibration Due"=w194) -> (w206:T7)
        n86 = call <vilib>:"Add State(s) to Queue__jki_lib_state_machine.vi"("State(s) in (\"\")"=w209) -> ("States Out"=w208:string)  [unwired: 14 in]
      }
      frame "Check Calibration Date" {
        # "Your code here.\n(You can make a copy of, or modify, this frame)"
        n87 = Unbundle By Name(w218) -> ("Calibration Due"=w210:T3, "Size"=w216:i32)
        n88 = for {
          N: w216 -> [_]
          tunnel: w210 -> [w227]
          tunnel: [w225] -> w215 mode=indexing
          i -> [w226]
          n89 = case shown="3" w226 {
            tunnel: w227 -> [w234 w241 w248 w255 w262 w269 w276 w283 w290 w297 w304 w311 w318 w325 w332 w339 w346 w353 w360 w367]
            tunnel: [w228 w235 w243 w249 w256 w263 w270 w277 w284 w291 w299 w306 w313 w319 w327 w334 w341 w348 w354 w361] -> w225
            frame 0, Default {
              n90 = Get Date/Time In Seconds() -> (seconds since 1Jan1904=w233:timestamp)
              n91 = Unbundle By Name(w234) -> ("Eq1"=w232:timestamp)
              n92 = Get Date/Time String(seconds (now)=w233) -> (date string=w231:string)  [unwired: 2 in, 1 out]
              n93 = Get Date/Time String(seconds (now)=w232) -> (date string=w230:string)  [unwired: 2 in, 1 out]
              n94 = call "UTILITY Date String Days.vi"("First date"=w231, "Second date"=w230) -> ("Elapsed days"=w229:i32)  [unwired: 8 in, 1 out]
              n95 = call "HEWH Check for Uninitialized Dates.vi"("date string"=w230, "Elapsed days in"=w229) -> ("Elapsed days out"=w228:i32)  [unwired: 9 in]
            }
            frame 1 {
              n96 = Unbundle By Name(w241) -> ("Eq2"=w238:timestamp)
              n97 = Get Date/Time In Seconds() -> (seconds since 1Jan1904=w240:timestamp)
              n98 = Get Date/Time String(seconds (now)=w240) -> (date string=w239:string)  [unwired: 2 in, 1 out]
              n99 = Get Date/Time String(seconds (now)=w238) -> (date string=w237:string)  [unwired: 2 in, 1 out]
              n100 = call "UTILITY Date String Days.vi"("First date"=w239, "Second date"=w237) -> ("Elapsed days"=w236:i32)  [unwired: 8 in, 1 out]
              n101 = call "HEWH Check for Uninitialized Dates.vi"("date string"=w237, "Elapsed days in"=w236) -> ("Elapsed days out"=w235:i32)  [unwired: 9 in]
            }
            frame 2 {
              n102 = Get Date/Time In Seconds() -> (seconds since 1Jan1904=w247:timestamp)
              n103 = Unbundle By Name(w248) -> ("Eq3"=w245:timestamp)
              n104 = Get Date/Time String(seconds (now)=w247) -> (date string=w246:string)  [unwired: 2 in, 1 out]
              n105 = Get Date/Time String(seconds (now)=w245) -> (date string=w242:string)  [unwired: 2 in, 1 out]
              n106 = call "UTILITY Date String Days.vi"("First date"=w246, "Second date"=w242) -> ("Elapsed days"=w244:i32)  [unwired: 8 in, 1 out]
              n107 = call "HEWH Check for Uninitialized Dates.vi"("date string"=w242, "Elapsed days in"=w244) -> ("Elapsed days out"=w243:i32)  [unwired: 9 in]
            }
            frame 3 {
              n108 = Get Date/Time In Seconds() -> (seconds since 1Jan1904=w254:timestamp)
              n109 = Unbundle By Name(w255) -> ("Eq4"=w252:timestamp)
              n110 = Get Date/Time String(seconds (now)=w254) -> (date string=w253:string)  [unwired: 2 in, 1 out]
              n111 = Get Date/Time String(seconds (now)=w252) -> (date string=w251:string)  [unwired: 2 in, 1 out]
              n112 = call "UTILITY Date String Days.vi"("First date"=w253, "Second date"=w251) -> ("Elapsed days"=w250:i32)  [unwired: 8 in, 1 out]
              n113 = call "HEWH Check for Uninitialized Dates.vi"("date string"=w251, "Elapsed days in"=w250) -> ("Elapsed days out"=w249:i32)  [unwired: 9 in]
            }
            frame 4 {
              n114 = Get Date/Time In Seconds() -> (seconds since 1Jan1904=w261:timestamp)
              n115 = Unbundle By Name(w262) -> ("Eq5"=w259:timestamp)
              n116 = Get Date/Time String(seconds (now)=w261) -> (date string=w260:string)  [unwired: 2 in, 1 out]
              n117 = Get Date/Time String(seconds (now)=w259) -> (date string=w258:string)  [unwired: 2 in, 1 out]
              n118 = call "UTILITY Date String Days.vi"("First date"=w260, "Second date"=w258) -> ("Elapsed days"=w257:i32)  [unwired: 8 in, 1 out]
              n119 = call "HEWH Check for Uninitialized Dates.vi"("date string"=w258, "Elapsed days in"=w257) -> ("Elapsed days out"=w256:i32)  [unwired: 9 in]
            }
            frame 5 {
              n120 = Get Date/Time In Seconds() -> (seconds since 1Jan1904=w268:timestamp)
              n121 = Unbundle By Name(w269) -> ("Eq6"=w266:timestamp)
              n122 = Get Date/Time String(seconds (now)=w268) -> (date string=w267:string)  [unwired: 2 in, 1 out]
              n123 = Get Date/Time String(seconds (now)=w266) -> (date string=w265:string)  [unwired: 2 in, 1 out]
              n124 = call "UTILITY Date String Days.vi"("First date"=w267, "Second date"=w265) -> ("Elapsed days"=w264:i32)  [unwired: 8 in, 1 out]
              n125 = call "HEWH Check for Uninitialized Dates.vi"("date string"=w265, "Elapsed days in"=w264) -> ("Elapsed days out"=w263:i32)  [unwired: 9 in]
            }
            frame 6 {
              n126 = Get Date/Time In Seconds() -> (seconds since 1Jan1904=w275:timestamp)
              n127 = Unbundle By Name(w276) -> ("Eq7"=w273:timestamp)
              n128 = Get Date/Time String(seconds (now)=w275) -> (date string=w274:string)  [unwired: 2 in, 1 out]
              n129 = Get Date/Time String(seconds (now)=w273) -> (date string=w272:string)  [unwired: 2 in, 1 out]
              n130 = call "UTILITY Date String Days.vi"("First date"=w274, "Second date"=w272) -> ("Elapsed days"=w271:i32)  [unwired: 8 in, 1 out]
              n131 = call "HEWH Check for Uninitialized Dates.vi"("date string"=w272, "Elapsed days in"=w271) -> ("Elapsed days out"=w270:i32)  [unwired: 9 in]
            }
            frame 7 {
              n132 = Get Date/Time In Seconds() -> (seconds since 1Jan1904=w282:timestamp)
              n133 = Get Date/Time String(seconds (now)=w282) -> (date string=w281:string)  [unwired: 2 in, 1 out]
              n134 = Unbundle By Name(w283) -> ("Eq8"=w280:timestamp)
              n135 = Get Date/Time String(seconds (now)=w280) -> (date string=w279:string)  [unwired: 2 in, 1 out]
              n136 = call "UTILITY Date String Days.vi"("First date"=w281, "Second date"=w279) -> ("Elapsed days"=w278:i32)  [unwired: 8 in, 1 out]
              n137 = call "HEWH Check for Uninitialized Dates.vi"("date string"=w279, "Elapsed days in"=w278) -> ("Elapsed days out"=w277:i32)  [unwired: 9 in]
            }
            frame 8 {
              n138 = Get Date/Time In Seconds() -> (seconds since 1Jan1904=w289:timestamp)
              n139 = Get Date/Time String(seconds (now)=w289) -> (date string=w288:string)  [unwired: 2 in, 1 out]
              n140 = Unbundle By Name(w290) -> ("Eq9"=w287:timestamp)
              n141 = Get Date/Time String(seconds (now)=w287) -> (date string=w286:string)  [unwired: 2 in, 1 out]
              n142 = call "UTILITY Date String Days.vi"("First date"=w288, "Second date"=w286) -> ("Elapsed days"=w285:i32)  [unwired: 8 in, 1 out]
              n143 = call "HEWH Check for Uninitialized Dates.vi"("date string"=w286, "Elapsed days in"=w285) -> ("Elapsed days out"=w284:i32)  [unwired: 9 in]
            }
            frame 9 {
              n144 = Get Date/Time In Seconds() -> (seconds since 1Jan1904=w296:timestamp)
              n145 = Get Date/Time String(seconds (now)=w296) -> (date string=w295:string)  [unwired: 2 in, 1 out]
              n146 = Unbundle By Name(w297) -> ("Eq10"=w294:timestamp)
              n147 = Get Date/Time String(seconds (now)=w294) -> (date string=w293:string)  [unwired: 2 in, 1 out]
              n148 = call "UTILITY Date String Days.vi"("First date"=w295, "Second date"=w293) -> ("Elapsed days"=w292:i32)  [unwired: 8 in, 1 out]
              n149 = call "HEWH Check for Uninitialized Dates.vi"("date string"=w293, "Elapsed days in"=w292) -> ("Elapsed days out"=w291:i32)  [unwired: 9 in]
            }
            frame 10 {
              n150 = Get Date/Time In Seconds() -> (seconds since 1Jan1904=w303:timestamp)
              n151 = Unbundle By Name(w304) -> ("Eq11"=w301:timestamp)
              n152 = Get Date/Time String(seconds (now)=w303) -> (date string=w302:string)  [unwired: 2 in, 1 out]
              n153 = Get Date/Time String(seconds (now)=w301) -> (date string=w298:string)  [unwired: 2 in, 1 out]
              n154 = call "UTILITY Date String Days.vi"("First date"=w302, "Second date"=w298) -> ("Elapsed days"=w300:i32)  [unwired: 8 in, 1 out]
              n155 = call "HEWH Check for Uninitialized Dates.vi"("date string"=w298, "Elapsed days in"=w300) -> ("Elapsed days out"=w299:i32)  [unwired: 9 in]
            }
            frame 11 {
              n156 = Get Date/Time In Seconds() -> (seconds since 1Jan1904=w310:timestamp)
              n157 = Get Date/Time String(seconds (now)=w310) -> (date string=w309:string)  [unwired: 2 in, 1 out]
              n158 = Unbundle By Name(w311) -> ("Eq12"=w308:timestamp)
              n159 = Get Date/Time String(seconds (now)=w308) -> (date string=w305:string)  [unwired: 2 in, 1 out]
              n160 = call "UTILITY Date String Days.vi"("First date"=w309, "Second date"=w305) -> ("Elapsed days"=w307:i32)  [unwired: 8 in, 1 out]
              n161 = call "HEWH Check for Uninitialized Dates.vi"("date string"=w305, "Elapsed days in"=w307) -> ("Elapsed days out"=w306:i32)  [unwired: 9 in]
            }
            frame 12 {
              n162 = Get Date/Time In Seconds() -> (seconds since 1Jan1904=w317:timestamp)
              n163 = Unbundle By Name(w318) -> ("Eq13"=w315:timestamp)
              n164 = Get Date/Time String(seconds (now)=w317) -> (date string=w316:string)  [unwired: 2 in, 1 out]
              n165 = Get Date/Time String(seconds (now)=w315) -> (date string=w312:string)  [unwired: 2 in, 1 out]
              n166 = call "UTILITY Date String Days.vi"("First date"=w316, "Second date"=w312) -> ("Elapsed days"=w314:i32)  [unwired: 8 in, 1 out]
              n167 = call "HEWH Check for Uninitialized Dates.vi"("date string"=w312, "Elapsed days in"=w314) -> ("Elapsed days out"=w313:i32)  [unwired: 9 in]
            }
            frame 13 {
              n168 = Get Date/Time In Seconds() -> (seconds since 1Jan1904=w324:timestamp)
              n169 = Unbundle By Name(w325) -> ("Eq14"=w322:timestamp)
              n170 = Get Date/Time String(seconds (now)=w324) -> (date string=w323:string)  [unwired: 2 in, 1 out]
              n171 = Get Date/Time String(seconds (now)=w322) -> (date string=w321:string)  [unwired: 2 in, 1 out]
              n172 = call "UTILITY Date String Days.vi"("First date"=w323, "Second date"=w321) -> ("Elapsed days"=w320:i32)  [unwired: 8 in, 1 out]
              n173 = call "HEWH Check for Uninitialized Dates.vi"("date string"=w321, "Elapsed days in"=w320) -> ("Elapsed days out"=w319:i32)  [unwired: 9 in]
            }
            frame 14 {
              n174 = Get Date/Time In Seconds() -> (seconds since 1Jan1904=w331:timestamp)
              n175 = Get Date/Time String(seconds (now)=w331) -> (date string=w330:string)  [unwired: 2 in, 1 out]
              n176 = Unbundle By Name(w332) -> ("Eq15"=w329:timestamp)
              n177 = Get Date/Time String(seconds (now)=w329) -> (date string=w326:string)  [unwired: 2 in, 1 out]
              n178 = call "UTILITY Date String Days.vi"("First date"=w330, "Second date"=w326) -> ("Elapsed days"=w328:i32)  [unwired: 8 in, 1 out]
              n179 = call "HEWH Check for Uninitialized Dates.vi"("date string"=w326, "Elapsed days in"=w328) -> ("Elapsed days out"=w327:i32)  [unwired: 9 in]
            }
            frame 15 {
              n180 = Get Date/Time In Seconds() -> (seconds since 1Jan1904=w338:timestamp)
              n181 = Unbundle By Name(w339) -> ("Eq16"=w336:timestamp)
              n182 = Get Date/Time String(seconds (now)=w338) -> (date string=w337:string)  [unwired: 2 in, 1 out]
              n183 = Get Date/Time String(seconds (now)=w336) -> (date string=w333:string)  [unwired: 2 in, 1 out]
              n184 = call "UTILITY Date String Days.vi"("First date"=w337, "Second date"=w333) -> ("Elapsed days"=w335:i32)  [unwired: 8 in, 1 out]
              n185 = call "HEWH Check for Uninitialized Dates.vi"("date string"=w333, "Elapsed days in"=w335) -> ("Elapsed days out"=w334:i32)  [unwired: 9 in]
            }
            frame 16 {
              n186 = Get Date/Time In Seconds() -> (seconds since 1Jan1904=w345:timestamp)
              n187 = Unbundle By Name(w346) -> ("Eq17"=w343:timestamp)
              n188 = Get Date/Time String(seconds (now)=w345) -> (date string=w344:string)  [unwired: 2 in, 1 out]
              n189 = Get Date/Time String(seconds (now)=w343) -> (date string=w340:string)  [unwired: 2 in, 1 out]
              n190 = call "UTILITY Date String Days.vi"("First date"=w344, "Second date"=w340) -> ("Elapsed days"=w342:i32)  [unwired: 8 in, 1 out]
              n191 = call "HEWH Check for Uninitialized Dates.vi"("date string"=w340, "Elapsed days in"=w342) -> ("Elapsed days out"=w341:i32)  [unwired: 9 in]
            }
            frame 17 {
              n192 = Unbundle By Name(w353) -> ("Eq18"=w350:timestamp)
              n193 = Get Date/Time In Seconds() -> (seconds since 1Jan1904=w352:timestamp)
              n194 = Get Date/Time String(seconds (now)=w352) -> (date string=w351:string)  [unwired: 2 in, 1 out]
              n195 = Get Date/Time String(seconds (now)=w350) -> (date string=w347:string)  [unwired: 2 in, 1 out]
              n196 = call "UTILITY Date String Days.vi"("First date"=w351, "Second date"=w347) -> ("Elapsed days"=w349:i32)  [unwired: 8 in, 1 out]
              n197 = call "HEWH Check for Uninitialized Dates.vi"("date string"=w347, "Elapsed days in"=w349) -> ("Elapsed days out"=w348:i32)  [unwired: 9 in]
            }
            frame 18 {
              n198 = Get Date/Time In Seconds() -> (seconds since 1Jan1904=w359:timestamp)
              n199 = Unbundle By Name(w360) -> ("Eq19"=w357:timestamp)
              n200 = Get Date/Time String(seconds (now)=w359) -> (date string=w358:string)  [unwired: 2 in, 1 out]
              n201 = Get Date/Time String(seconds (now)=w357) -> (date string=w356:string)  [unwired: 2 in, 1 out]
              n202 = call "UTILITY Date String Days.vi"("First date"=w358, "Second date"=w356) -> ("Elapsed days"=w355:i32)  [unwired: 8 in, 1 out]
              n203 = call "HEWH Check for Uninitialized Dates.vi"("date string"=w356, "Elapsed days in"=w355) -> ("Elapsed days out"=w354:i32)  [unwired: 9 in]
            }
            frame 19 {
              n204 = Get Date/Time In Seconds() -> (seconds since 1Jan1904=w366:timestamp)
              n205 = Unbundle By Name(w367) -> ("Eq20"=w364:timestamp)
              n206 = Get Date/Time String(seconds (now)=w366) -> (date string=w365:string)  [unwired: 2 in, 1 out]
              n207 = Get Date/Time String(seconds (now)=w364) -> (date string=w363:string)  [unwired: 2 in, 1 out]
              n208 = call "UTILITY Date String Days.vi"("First date"=w365, "Second date"=w363) -> ("Elapsed days"=w362:i32)  [unwired: 8 in, 1 out]
              n209 = call "HEWH Check for Uninitialized Dates.vi"("date string"=w363, "Elapsed days in"=w362) -> ("Elapsed days out"=w361:i32)  [unwired: 9 in]
            }
          }
        }
        n210 = Array Max & Min(array=w215) -> (min value=w212:i32)  [unwired: 3 out]
        n211 = Less?(x=w212, y=30) -> (x < y?=w213:bool)
        n212 = Number To Decimal String(number=w212) -> (decimal integer string=w211:string)  [unwired: 1 in]
        n213 = case shown="True" w213 {
          tunnel: w211 -> [_ w224]
          frame False {
          }
          frame True {
            n214 = Concatenate Strings("Componets will be out of calibration in " ("message"), w224, " Days" ("string")) -> (w221:string)
            "concatenated string" <- w221
            n215 = One Button Dialog(message=w221) -> ()  [unwired: 1 in, 1 out]
          }
        }
        n216 = call <vilib>:"Add State(s) to Queue__jki_lib_state_machine.vi"("State(s) in (\"\")"=w220) -> ("States Out"=w219:string)  [unwired: 14 in]
      }
      frame "Equipment Desc" {
        # "Your code here.\n(You can make a copy of, or modify, this frame)"
        n217 = Unbundle By Name(w375) -> ("Equipment Description"=w373:T1, "Total Array"=w372:string[][])
        n218 = for {
          N: 20 -> [_]
          tunnel: w373 -> [w387]
          tunnel: string[] [] -> [w385]
          tunnel: [w384] -> w370 mode=indexing
          tunnel: [w383] -> w376
          tunnel: w377 -> [w383]
          i -> [w386]
          n219 = case shown="15" w386 {
            tunnel: w387 -> [w389 w391 w393 w395 w397 w399 w401 w403 w405 w407 w409 w411 w413 w415 w417 w419 w421 w422 w425 w427]
            tunnel: [w388 w390 w392 w394 w396 w398 w400 w402 w404 w406 w408 w410 w412 w414 w416 w418 w420 w423 w424 w426] -> w382
            frame 0, Default {
              n220 = Unbundle By Name(w389) -> ("Eq 1"=w388:string)
            }
            frame 1 {
              n221 = Unbundle By Name(w391) -> ("Eq 2"=w390:string)
            }
            frame 2 {
              n222 = Unbundle By Name(w393) -> ("Eq 3"=w392:string)
            }
            frame 3 {
              n223 = Unbundle By Name(w395) -> ("Eq 4"=w394:string)
            }
            frame 4 {
              n224 = Unbundle By Name(w397) -> ("Eq 5"=w396:string)
            }
            frame 5 {
              n225 = Unbundle By Name(w399) -> ("Eq 6"=w398:string)
            }
            frame 6 {
              n226 = Unbundle By Name(w401) -> ("Eq 7"=w400:string)
            }
            frame 7 {
              n227 = Unbundle By Name(w403) -> ("Eq 8"=w402:string)
            }
            frame 8 {
              n228 = Unbundle By Name(w405) -> ("Eq 9"=w404:string)
            }
            frame 9 {
              n229 = Unbundle By Name(w407) -> ("Eq 10"=w406:string)
            }
            frame 10 {
              n230 = Unbundle By Name(w409) -> ("Eq 11"=w408:string)
            }
            frame 11 {
              n231 = Unbundle By Name(w411) -> ("Eq 12"=w410:string)
            }
            frame 12 {
              n232 = Unbundle By Name(w413) -> ("Eq 13"=w412:string)
            }
            frame 13 {
              n233 = Unbundle By Name(w415) -> ("Eq 14"=w414:string)
            }
            frame 14 {
              n234 = Unbundle By Name(w417) -> ("Eq 15"=w416:string)
            }
            frame 15 {
              n235 = Unbundle By Name(w419) -> ("Eq 16"=w418:string)
            }
            frame 16 {
              n236 = Unbundle By Name(w421) -> ("Eq 17"=w420:string)
            }
            frame 17 {
              n237 = Unbundle By Name(w422) -> ("Eq 18"=w423:string)
            }
            frame 18 {
              n238 = Unbundle By Name(w425) -> ("Eq 19"=w424:string)
            }
            frame 19 {
              n239 = Unbundle By Name(w427) -> ("Eq 20"=w426:string)
            }
          }
          n240 = Build Array (concatenate)(w385, w382) -> (w384:string[])
        }
        n241 = call "UTILITY Array Get 1D String Column From 2D.vi"("2D Array Data"=w370, "column index"=0) -> ("Column Data"=w368:string[])  [unwired: 13 in]
        n242 = Build Array (concatenate)(w372, w368) -> (w371:string[][])
        n243 = Bundle By Name(cluster=w375, "Total Array"=w371) -> (w374:T7)
        n244 = call <vilib>:"Add State(s) to Queue__jki_lib_state_machine.vi"("State(s) in (\"\")"=w381) -> ("States Out"=w380:string)  [unwired: 14 in]
      }
      frame "Manufacturer" {
        # "Your code here.\n(You can make a copy of, or modify, this frame)"
        n245 = Unbundle By Name(w435) -> ("Manufacturer"=w433:T1, "Total Array"=w432:string[][])
        n246 = for {
          N: 20 -> [_]
          tunnel: w433 -> [w447]
          tunnel: string[] [] -> [w445]
          tunnel: [w444] -> w430 mode=indexing
          tunnel: [w443] -> w436
          tunnel: w437 -> [w443]
          i -> [w446]
          n247 = case shown="15" w446 {
            tunnel: w447 -> [w449 w451 w453 w455 w457 w459 w461 w463 w465 w467 w469 w471 w473 w475 w477 w479 w481 w482 w485 w487]
            tunnel: [w448 w450 w452 w454 w456 w458 w460 w462 w464 w466 w468 w470 w472 w474 w476 w478 w480 w483 w484 w486] -> w442
            frame 0, Default {
              n248 = Unbundle By Name(w449) -> ("Eq 1"=w448:string)
            }
            frame 1 {
              n249 = Unbundle By Name(w451) -> ("Eq 2"=w450:string)
            }
            frame 2 {
              n250 = Unbundle By Name(w453) -> ("Eq 3"=w452:string)
            }
            frame 3 {
              n251 = Unbundle By Name(w455) -> ("Eq 4"=w454:string)
            }
            frame 4 {
              n252 = Unbundle By Name(w457) -> ("Eq 5"=w456:string)
            }
            frame 5 {
              n253 = Unbundle By Name(w459) -> ("Eq 6"=w458:string)
            }
            frame 6 {
              n254 = Unbundle By Name(w461) -> ("Eq 7"=w460:string)
            }
            frame 7 {
              n255 = Unbundle By Name(w463) -> ("Eq 8"=w462:string)
            }
            frame 8 {
              n256 = Unbundle By Name(w465) -> ("Eq 9"=w464:string)
            }
            frame 9 {
              n257 = Unbundle By Name(w467) -> ("Eq 10"=w466:string)
            }
            frame 10 {
              n258 = Unbundle By Name(w469) -> ("Eq 11"=w468:string)
            }
            frame 11 {
              n259 = Unbundle By Name(w471) -> ("Eq 12"=w470:string)
            }
            frame 12 {
              n260 = Unbundle By Name(w473) -> ("Eq 13"=w472:string)
            }
            frame 13 {
              n261 = Unbundle By Name(w475) -> ("Eq 14"=w474:string)
            }
            frame 14 {
              n262 = Unbundle By Name(w477) -> ("Eq 15"=w476:string)
            }
            frame 15 {
              n263 = Unbundle By Name(w479) -> ("Eq 16"=w478:string)
            }
            frame 16 {
              n264 = Unbundle By Name(w481) -> ("Eq 17"=w480:string)
            }
            frame 17 {
              n265 = Unbundle By Name(w482) -> ("Eq 18"=w483:string)
            }
            frame 18 {
              n266 = Unbundle By Name(w485) -> ("Eq 19"=w484:string)
            }
            frame 19 {
              n267 = Unbundle By Name(w487) -> ("Eq 20"=w486:string)
            }
          }
          n268 = Build Array (concatenate)(w445, w442) -> (w444:string[])
        }
        n269 = call "UTILITY Array Get 1D String Column From 2D.vi"("2D Array Data"=w430, "column index"=0) -> ("Column Data"=w428:string[])  [unwired: 13 in]
        n270 = Build Array (concatenate)(w432, w428) -> (w431:string[][])
        n271 = Bundle By Name(cluster=w435, "Total Array"=w431) -> (w434:T7)
        n272 = call <vilib>:"Add State(s) to Queue__jki_lib_state_machine.vi"("State(s) in (\"\")"=w441) -> ("States Out"=w440:string)  [unwired: 14 in]
      }
      frame "Model Number" {
        # "Your code here.\n(You can make a copy of, or modify, this frame)"
        n273 = Unbundle By Name(w495) -> ("Model Number"=w493:T1, "Total Array"=w492:string[][])
        n274 = for {
          N: 20 -> [_]
          tunnel: w493 -> [w507]
          tunnel: string[] [] -> [w505]
          tunnel: [w504] -> w490 mode=indexing
          tunnel: [w503] -> w496
          tunnel: w497 -> [w503]
          i -> [w506]
          n275 = case shown="15" w506 {
            tunnel: w507 -> [w509 w511 w513 w515 w517 w519 w521 w523 w525 w527 w529 w531 w533 w535 w537 w539 w541 w542 w545 w547]
            tunnel: [w508 w510 w512 w514 w516 w518 w520 w522 w524 w526 w528 w530 w532 w534 w536 w538 w540 w543 w544 w546] -> w502
            frame 0, Default {
              n276 = Unbundle By Name(w509) -> ("Eq 1"=w508:string)
            }
            frame 1 {
              n277 = Unbundle By Name(w511) -> ("Eq 2"=w510:string)
            }
            frame 2 {
              n278 = Unbundle By Name(w513) -> ("Eq 3"=w512:string)
            }
            frame 3 {
              n279 = Unbundle By Name(w515) -> ("Eq 4"=w514:string)
            }
            frame 4 {
              n280 = Unbundle By Name(w517) -> ("Eq 5"=w516:string)
            }
            frame 5 {
              n281 = Unbundle By Name(w519) -> ("Eq 6"=w518:string)
            }
            frame 6 {
              n282 = Unbundle By Name(w521) -> ("Eq 7"=w520:string)
            }
            frame 7 {
              n283 = Unbundle By Name(w523) -> ("Eq 8"=w522:string)
            }
            frame 8 {
              n284 = Unbundle By Name(w525) -> ("Eq 9"=w524:string)
            }
            frame 9 {
              n285 = Unbundle By Name(w527) -> ("Eq 10"=w526:string)
            }
            frame 10 {
              n286 = Unbundle By Name(w529) -> ("Eq 11"=w528:string)
            }
            frame 11 {
              n287 = Unbundle By Name(w531) -> ("Eq 12"=w530:string)
            }
            frame 12 {
              n288 = Unbundle By Name(w533) -> ("Eq 13"=w532:string)
            }
            frame 13 {
              n289 = Unbundle By Name(w535) -> ("Eq 14"=w534:string)
            }
            frame 14 {
              n290 = Unbundle By Name(w537) -> ("Eq 15"=w536:string)
            }
            frame 15 {
              n291 = Unbundle By Name(w539) -> ("Eq 16"=w538:string)
            }
            frame 16 {
              n292 = Unbundle By Name(w541) -> ("Eq 17"=w540:string)
            }
            frame 17 {
              n293 = Unbundle By Name(w542) -> ("Eq 18"=w543:string)
            }
            frame 18 {
              n294 = Unbundle By Name(w545) -> ("Eq 19"=w544:string)
            }
            frame 19 {
              n295 = Unbundle By Name(w547) -> ("Eq 20"=w546:string)
            }
          }
          n296 = Build Array (concatenate)(w505, w502) -> (w504:string[])
        }
        n297 = call "UTILITY Array Get 1D String Column From 2D.vi"("2D Array Data"=w490, "column index"=0) -> ("Column Data"=w488:string[])  [unwired: 13 in]
        n298 = Build Array (concatenate)(w492, w488) -> (w491:string[][])
        n299 = Bundle By Name(cluster=w495, "Total Array"=w491) -> (w494:T7)
        n300 = call <vilib>:"Add State(s) to Queue__jki_lib_state_machine.vi"("State(s) in (\"\")"=w501) -> ("States Out"=w500:string)  [unwired: 14 in]
      }
      frame "Write Calibration ID" {
        # "Your code here.\n(You can make a copy of, or modify, this frame)"
        n301 = Unbundle By Name(w555) -> ("Calibration ID"=w553:T1, "Total Array"=w552:string[][])
        n302 = for {
          N: 20 -> [_]
          tunnel: w553 -> [w567]
          tunnel: string[] [] -> [w565]
          tunnel: [w564] -> w550 mode=indexing
          tunnel: [w563] -> w556
          tunnel: w557 -> [w563]
          i -> [w566]
          n303 = case shown="15" w566 {
            tunnel: w567 -> [w569 w571 w573 w575 w577 w579 w581 w583 w585 w587 w589 w591 w593 w595 w597 w599 w601 w602 w605 w607]
            tunnel: [w568 w570 w572 w574 w576 w578 w580 w582 w584 w586 w588 w590 w592 w594 w596 w598 w600 w603 w604 w606] -> w562
            frame 0, Default {
              n304 = Unbundle By Name(w569) -> ("Eq 1"=w568:string)
            }
            frame 1 {
              n305 = Unbundle By Name(w571) -> ("Eq 2"=w570:string)
            }
            frame 2 {
              n306 = Unbundle By Name(w573) -> ("Eq 3"=w572:string)
            }
            frame 3 {
              n307 = Unbundle By Name(w575) -> ("Eq 4"=w574:string)
            }
            frame 4 {
              n308 = Unbundle By Name(w577) -> ("Eq 5"=w576:string)
            }
            frame 5 {
              n309 = Unbundle By Name(w579) -> ("Eq 6"=w578:string)
            }
            frame 6 {
              n310 = Unbundle By Name(w581) -> ("Eq 7"=w580:string)
            }
            frame 7 {
              n311 = Unbundle By Name(w583) -> ("Eq 8"=w582:string)
            }
            frame 8 {
              n312 = Unbundle By Name(w585) -> ("Eq 9"=w584:string)
            }
            frame 9 {
              n313 = Unbundle By Name(w587) -> ("Eq 10"=w586:string)
            }
            frame 10 {
              n314 = Unbundle By Name(w589) -> ("Eq 11"=w588:string)
            }
            frame 11 {
              n315 = Unbundle By Name(w591) -> ("Eq 12"=w590:string)
            }
            frame 12 {
              n316 = Unbundle By Name(w593) -> ("Eq 13"=w592:string)
            }
            frame 13 {
              n317 = Unbundle By Name(w595) -> ("Eq 14"=w594:string)
            }
            frame 14 {
              n318 = Unbundle By Name(w597) -> ("Eq 15"=w596:string)
            }
            frame 15 {
              n319 = Unbundle By Name(w599) -> ("Eq 16"=w598:string)
            }
            frame 16 {
              n320 = Unbundle By Name(w601) -> ("Eq 17"=w600:string)
            }
            frame 17 {
              n321 = Unbundle By Name(w602) -> ("Eq 18"=w603:string)
            }
            frame 18 {
              n322 = Unbundle By Name(w605) -> ("Eq 19"=w604:string)
            }
            frame 19 {
              n323 = Unbundle By Name(w607) -> ("Eq 20"=w606:string)
            }
          }
          n324 = Build Array (concatenate)(w565, w562) -> (w564:string[])
        }
        n325 = call "UTILITY Array Get 1D String Column From 2D.vi"("2D Array Data"=w550, "column index"=0) -> ("Column Data"=w548:string[])  [unwired: 13 in]
        n326 = Build Array (concatenate)(w552, w548) -> (w551:string[][])
        n327 = Bundle By Name(cluster=w555, "Total Array"=w551) -> (w554:T7)
        n328 = call <vilib>:"Add State(s) to Queue__jki_lib_state_machine.vi"("State(s) in (\"\")"=w561) -> ("States Out"=w560:string)  [unwired: 14 in]
      }
      frame "Write Calibration SN" {
        n329 = Unbundle By Name(w615) -> ("Serial Number"=w613:T2, "Total Array"=w612:string[][])
        n330 = for {
          N: 20 -> [_]
          tunnel: w613 -> [w627]
          tunnel: string[] [] -> [w625]
          tunnel: [w624] -> w610 mode=indexing
          tunnel: [w623] -> w616
          tunnel: w617 -> [w623]
          i -> [w626]
          n331 = case shown="15" w626 {
            tunnel: w627 -> [w629 w631 w633 w635 w637 w639 w641 w643 w645 w647 w649 w651 w653 w655 w657 w659 w661 w663 w665 w667]
            tunnel: [w628 w630 w632 w634 w636 w638 w640 w642 w644 w646 w648 w650 w652 w654 w656 w658 w660 w662 w664 w666] -> w622
            frame 0, Default {
              n332 = Unbundle By Name(w629) -> ("Eq 1"=w628:string)
            }
            frame 1 {
              n333 = Unbundle By Name(w631) -> ("Eq 2"=w630:string)
            }
            frame 2 {
              n334 = Unbundle By Name(w633) -> ("Eq 3"=w632:string)
            }
            frame 3 {
              n335 = Unbundle By Name(w635) -> ("Eq 4"=w634:string)
            }
            frame 4 {
              n336 = Unbundle By Name(w637) -> ("Eq 5"=w636:string)
            }
            frame 5 {
              n337 = Unbundle By Name(w639) -> ("Eq 6"=w638:string)
            }
            frame 6 {
              n338 = Unbundle By Name(w641) -> ("Eq 7"=w640:string)
            }
            frame 7 {
              n339 = Unbundle By Name(w643) -> ("Eq 8"=w642:string)
            }
            frame 8 {
              n340 = Unbundle By Name(w645) -> ("Eq 9"=w644:string)
            }
            frame 9 {
              n341 = Unbundle By Name(w647) -> ("Eq 10"=w646:string)
            }
            frame 10 {
              n342 = Unbundle By Name(w649) -> ("Eq 11"=w648:string)
            }
            frame 11 {
              n343 = Unbundle By Name(w651) -> ("Eq 12"=w650:string)
            }
            frame 12 {
              n344 = Unbundle By Name(w653) -> ("Eq 13"=w652:string)
            }
            frame 13 {
              n345 = Unbundle By Name(w655) -> ("Eq 14"=w654:string)
            }
            frame 14 {
              n346 = Unbundle By Name(w657) -> ("Eq 15"=w656:string)
            }
            frame 15 {
              n347 = Unbundle By Name(w659) -> ("Eq 16"=w658:string)
            }
            frame 16 {
              n348 = Unbundle By Name(w661) -> ("Eq 17"=w660:string)
            }
            frame 17 {
              n349 = Unbundle By Name(w663) -> ("Eq 18"=w662:string)
            }
            frame 18 {
              n350 = Unbundle By Name(w665) -> ("Eq 19"=w664:string)
            }
            frame 19 {
              n351 = Unbundle By Name(w667) -> ("Eq 20"=w666:string)
            }
          }
          n352 = Build Array (concatenate)(w625, w622) -> (w624:string[])
        }
        n353 = call "UTILITY Array Get 1D String Column From 2D.vi"("2D Array Data"=w610, "column index"=0) -> ("Column Data"=w608:string[])  [unwired: 13 in]
        "snta" <- w608
        n354 = Build Array (concatenate)(w612, w608) -> (w611:string[][])
        n355 = Bundle By Name(cluster=w615, "Total Array"=w611) -> (w614:T7)
        n356 = call <vilib>:"Add State(s) to Queue__jki_lib_state_machine.vi"("State(s) in (\"\")"=w621) -> ("States Out"=w620:string)  [unwired: 14 in]
      }
      frame "Last Calibration" {
        n357 = Unbundle By Name(w674) -> ("Last Calibrated"=w675:T3, "Total Array"=w670:string[][])
        n358 = for {
          N: 20 -> [_]
          tunnel: w675 -> [w689]
          tunnel: string[] [] -> [w687]
          tunnel: [w686] -> w672 mode=indexing
          tunnel: [w682] -> w676
          tunnel: w677 -> [w682]
          i -> [w688]
          n359 = case shown="0, Default" w688 {
            tunnel: w689 -> [w692 w695 w698 w701 w704 w707 w710 w713 w716 w719 w722 w725 w728 w731 w734 w737 w740 w743 w745 w749]
            tunnel: [w690 w693 w696 w699 w702 w705 w708 w711 w714 w717 w720 w723 w726 w729 w732 w735 w738 w741 w746 w747] -> w685
            frame 0, Default {
              n360 = Unbundle By Name(w692) -> ("Eq1"=w691:timestamp)
              n361 = Format Date/Time String(seconds (now)=w691) -> (date/time string=w690:string)  [unwired: 2 in]
            }
            frame 1 {
              n362 = Unbundle By Name(w695) -> ("Eq2"=w694:timestamp)
              n363 = Format Date/Time String(seconds (now)=w694) -> (date/time string=w693:string)  [unwired: 2 in]
            }
            frame 2 {
              n364 = Unbundle By Name(w698) -> ("Eq3"=w697:timestamp)
              n365 = Format Date/Time String(seconds (now)=w697) -> (date/time string=w696:string)  [unwired: 2 in]
            }
            frame 3 {
              n366 = Unbundle By Name(w701) -> ("Eq4"=w700:timestamp)
              n367 = Format Date/Time String(seconds (now)=w700) -> (date/time string=w699:string)  [unwired: 2 in]
            }
            frame 4 {
              n368 = Unbundle By Name(w704) -> ("Eq5"=w703:timestamp)
              n369 = Format Date/Time String(seconds (now)=w703) -> (date/time string=w702:string)  [unwired: 2 in]
            }
            frame 5 {
              n370 = Unbundle By Name(w707) -> ("Eq6"=w706:timestamp)
              n371 = Format Date/Time String(seconds (now)=w706) -> (date/time string=w705:string)  [unwired: 2 in]
            }
            frame 6 {
              n372 = Unbundle By Name(w710) -> ("Eq7"=w709:timestamp)
              n373 = Format Date/Time String(seconds (now)=w709) -> (date/time string=w708:string)  [unwired: 2 in]
            }
            frame 7 {
              n374 = Unbundle By Name(w713) -> ("Eq8"=w712:timestamp)
              n375 = Format Date/Time String(seconds (now)=w712) -> (date/time string=w711:string)  [unwired: 2 in]
            }
            frame 8 {
              n376 = Unbundle By Name(w716) -> ("Eq9"=w715:timestamp)
              n377 = Format Date/Time String(seconds (now)=w715) -> (date/time string=w714:string)  [unwired: 2 in]
            }
            frame 9 {
              n378 = Unbundle By Name(w719) -> ("Eq10"=w718:timestamp)
              n379 = Format Date/Time String(seconds (now)=w718) -> (date/time string=w717:string)  [unwired: 2 in]
            }
            frame 10 {
              n380 = Unbundle By Name(w722) -> ("Eq11"=w721:timestamp)
              n381 = Format Date/Time String(seconds (now)=w721) -> (date/time string=w720:string)  [unwired: 2 in]
            }
            frame 11 {
              n382 = Unbundle By Name(w725) -> ("Eq12"=w724:timestamp)
              n383 = Format Date/Time String(seconds (now)=w724) -> (date/time string=w723:string)  [unwired: 2 in]
            }
            frame 12 {
              n384 = Unbundle By Name(w728) -> ("Eq13"=w727:timestamp)
              n385 = Format Date/Time String(seconds (now)=w727) -> (date/time string=w726:string)  [unwired: 2 in]
            }
            frame 13 {
              n386 = Unbundle By Name(w731) -> ("Eq14"=w730:timestamp)
              n387 = Format Date/Time String(seconds (now)=w730) -> (date/time string=w729:string)  [unwired: 2 in]
            }
            frame 14 {
              n388 = Unbundle By Name(w734) -> ("Eq15"=w733:timestamp)
              n389 = Format Date/Time String(seconds (now)=w733) -> (date/time string=w732:string)  [unwired: 2 in]
            }
            frame 15 {
              n390 = Unbundle By Name(w737) -> ("Eq16"=w736:timestamp)
              n391 = Format Date/Time String(seconds (now)=w736) -> (date/time string=w735:string)  [unwired: 2 in]
            }
            frame 16 {
              n392 = Unbundle By Name(w740) -> ("Eq17"=w739:timestamp)
              n393 = Format Date/Time String(seconds (now)=w739) -> (date/time string=w738:string)  [unwired: 2 in]
            }
            frame 17 {
              n394 = Unbundle By Name(w743) -> ("Eq18"=w742:timestamp)
              n395 = Format Date/Time String(seconds (now)=w742) -> (date/time string=w741:string)  [unwired: 2 in]
            }
            frame 18 {
              n396 = Unbundle By Name(w745) -> ("Eq19"=w744:timestamp)
              n397 = Format Date/Time String(seconds (now)=w744) -> (date/time string=w746:string)  [unwired: 2 in]
            }
            frame 19 {
              n398 = Unbundle By Name(w749) -> ("Eq20"=w748:timestamp)
              n399 = Format Date/Time String(seconds (now)=w748) -> (date/time string=w747:string)  [unwired: 2 in]
            }
          }
          n400 = call <vilib>:"Space Constant.vi"() -> ("String"=w683:string)
          n401 = Match Pattern(string=w685, regular expression=w683) -> (before substring=w684:string)  [unwired: 1 in, 3 out]
          n402 = Build Array (concatenate)(w687, w684) -> (w686:string[])
        }
        n403 = call "UTILITY Array Get 1D String Column From 2D.vi"("2D Array Data"=w672, "column index"=0) -> ("Column Data"=w669:string[])  [unwired: 13 in]
        n404 = Build Array (concatenate)(w670, w669) -> (w668:string[][])
        n405 = Bundle By Name(cluster=w674, "Total Array"=w668) -> (w673:T7)
        n406 = call <vilib>:"Add State(s) to Queue__jki_lib_state_machine.vi"("State(s) in (\"\")"=w681) -> ("States Out"=w680:string)  [unwired: 14 in]
      }
      frame "Write Calibration Date" {
        n407 = Unbundle By Name(w756) -> ("Calibration Due"=w757:T3, "Total Array"=w752:string[][])
        n408 = for {
          N: 20 -> [_]
          tunnel: w757 -> [w771]
          tunnel: string[] [] -> [w769]
          tunnel: [w768] -> w754 mode=indexing
          tunnel: [w764] -> w758
          tunnel: w759 -> [w764]
          i -> [w770]
          n409 = case shown="15" w770 {
            tunnel: w771 -> [w774 w777 w780 w783 w786 w789 w792 w795 w798 w801 w804 w807 w810 w813 w816 w819 w822 w825 w827 w831]
            tunnel: [w772 w775 w778 w781 w784 w787 w790 w793 w796 w799 w802 w805 w808 w811 w814 w817 w820 w823 w828 w829] -> w767
            frame 0, Default {
              n410 = Unbundle By Name(w774) -> ("Eq1"=w773:timestamp)
              n411 = Format Date/Time String(seconds (now)=w773) -> (date/time string=w772:string)  [unwired: 2 in]
            }
            frame 1 {
              n412 = Unbundle By Name(w777) -> ("Eq2"=w776:timestamp)
              n413 = Format Date/Time String(seconds (now)=w776) -> (date/time string=w775:string)  [unwired: 2 in]
            }
            frame 2 {
              n414 = Unbundle By Name(w780) -> ("Eq3"=w779:timestamp)
              n415 = Format Date/Time String(seconds (now)=w779) -> (date/time string=w778:string)  [unwired: 2 in]
            }
            frame 3 {
              n416 = Unbundle By Name(w783) -> ("Eq4"=w782:timestamp)
              n417 = Format Date/Time String(seconds (now)=w782) -> (date/time string=w781:string)  [unwired: 2 in]
            }
            frame 4 {
              n418 = Unbundle By Name(w786) -> ("Eq5"=w785:timestamp)
              n419 = Format Date/Time String(seconds (now)=w785) -> (date/time string=w784:string)  [unwired: 2 in]
            }
            frame 5 {
              n420 = Unbundle By Name(w789) -> ("Eq6"=w788:timestamp)
              n421 = Format Date/Time String(seconds (now)=w788) -> (date/time string=w787:string)  [unwired: 2 in]
            }
            frame 6 {
              n422 = Unbundle By Name(w792) -> ("Eq7"=w791:timestamp)
              n423 = Format Date/Time String(seconds (now)=w791) -> (date/time string=w790:string)  [unwired: 2 in]
            }
            frame 7 {
              n424 = Unbundle By Name(w795) -> ("Eq8"=w794:timestamp)
              n425 = Format Date/Time String(seconds (now)=w794) -> (date/time string=w793:string)  [unwired: 2 in]
            }
            frame 8 {
              n426 = Unbundle By Name(w798) -> ("Eq9"=w797:timestamp)
              n427 = Format Date/Time String(seconds (now)=w797) -> (date/time string=w796:string)  [unwired: 2 in]
            }
            frame 9 {
              n428 = Unbundle By Name(w801) -> ("Eq10"=w800:timestamp)
              n429 = Format Date/Time String(seconds (now)=w800) -> (date/time string=w799:string)  [unwired: 2 in]
            }
            frame 10 {
              n430 = Unbundle By Name(w804) -> ("Eq11"=w803:timestamp)
              n431 = Format Date/Time String(seconds (now)=w803) -> (date/time string=w802:string)  [unwired: 2 in]
            }
            frame 11 {
              n432 = Unbundle By Name(w807) -> ("Eq12"=w806:timestamp)
              n433 = Format Date/Time String(seconds (now)=w806) -> (date/time string=w805:string)  [unwired: 2 in]
            }
            frame 12 {
              n434 = Unbundle By Name(w810) -> ("Eq13"=w809:timestamp)
              n435 = Format Date/Time String(seconds (now)=w809) -> (date/time string=w808:string)  [unwired: 2 in]
            }
            frame 13 {
              n436 = Unbundle By Name(w813) -> ("Eq14"=w812:timestamp)
              n437 = Format Date/Time String(seconds (now)=w812) -> (date/time string=w811:string)  [unwired: 2 in]
            }
            frame 14 {
              n438 = Unbundle By Name(w816) -> ("Eq15"=w815:timestamp)
              n439 = Format Date/Time String(seconds (now)=w815) -> (date/time string=w814:string)  [unwired: 2 in]
            }
            frame 15 {
              n440 = Unbundle By Name(w819) -> ("Eq16"=w818:timestamp)
              n441 = Format Date/Time String(seconds (now)=w818) -> (date/time string=w817:string)  [unwired: 2 in]
            }
            frame 16 {
              n442 = Unbundle By Name(w822) -> ("Eq17"=w821:timestamp)
              n443 = Format Date/Time String(seconds (now)=w821) -> (date/time string=w820:string)  [unwired: 2 in]
            }
            frame 17 {
              n444 = Unbundle By Name(w825) -> ("Eq18"=w824:timestamp)
              n445 = Format Date/Time String(seconds (now)=w824) -> (date/time string=w823:string)  [unwired: 2 in]
            }
            frame 18 {
              n446 = Unbundle By Name(w827) -> ("Eq19"=w826:timestamp)
              n447 = Format Date/Time String(seconds (now)=w826) -> (date/time string=w828:string)  [unwired: 2 in]
            }
            frame 19 {
              n448 = Unbundle By Name(w831) -> ("Eq20"=w830:timestamp)
              n449 = Format Date/Time String(seconds (now)=w830) -> (date/time string=w829:string)  [unwired: 2 in]
            }
          }
          n450 = call <vilib>:"Space Constant.vi"() -> ("String"=w765:string)
          n451 = Match Pattern(string=w767, regular expression=w765) -> (before substring=w766:string)  [unwired: 1 in, 3 out]
          n452 = Build Array (concatenate)(w769, w766) -> (w768:string[])
        }
        n453 = call "UTILITY Array Get 1D String Column From 2D.vi"("2D Array Data"=w754, "column index"=0) -> ("Column Data"=w751:string[])  [unwired: 13 in]
        n454 = Build Array (concatenate)(w752, w751) -> (w750:string[][])
        n455 = Bundle By Name(cluster=w756, "Total Array"=w750) -> (w755:T7)
        n456 = call <vilib>:"Add State(s) to Queue__jki_lib_state_machine.vi"("State(s) in (\"\")"=w763) -> ("States Out"=w762:string)  [unwired: 14 in]
      }
      frame "Write to File" {
        n457 = Unbundle By Name(w839) -> ("file path (dialog if empty)"=w838:path, "Total Array"=w835:string[][])
        n458 = Transpose 2D Array(2D array=w835) -> (transposed array=w834:string[][])
        n459 = call "HEWH Calibration Delete Unused String Lines.vi"("Total Array"=w834) -> ("Output Array"=w832:string[][])  [unwired: 10 in]
        "OutputData" <- w832
        n460 = call-poly <vilib>:"Write To Spreadsheet File.vi"("delimiter (\\t)"="," ("delimiter (\\t)"), "append to file? (new file:F)"=FALSE ("Keep Refnum Open"), "2D data"=w832, "file path (dialog if empty)"=w838) -> ()  [unwired: 4 in, 1 out]
        n461 = call <vilib>:"Add State(s) to Queue__jki_lib_state_machine.vi"("State(s) in (\"\")"=w841) -> ("States Out"=w840:string)  [unwired: 14 in]
      }
    }
  }
  "error out" <- w2
